vi "0.Main.vi"() -> ()   [LabVIEW 2021]
uses:
  controls/initialise cluster.ctl
  controls/developer_test sequence.ctl
  controls/test step description.ctl
  controls/test type selection.ctl
  controls/comparison selection.ctl
  controls/DMM measuring state.ctl
  <vilib>/Utility/miscctls.llb/LVPointTypeDef.ctl
  support/Message Queue/Enqueue Message (Single).vi
  support/Message Queue/RMU Message Queue.lvlib
  support/User Event - Stop/RMU User Event - Stop.lvlib
  GPT-9800_GSB_L2011/GPT-9000.lvlib
panel:
  out "Output values":T1
  out "Varaint Selection":string
  out "Tempertaure Sensor":string
  out "Result":bool
  out "m second":u32
  out "Hillppot Comport":refnum<visa-resource-name>
  out "Final Weld Resistance Result":string
  out "Limits revision":string
  out "weld voltage":dbl[](array[numeric]) format="%#_6p"
  out "Test Start Time":string
  out "Result indicators":refnum<vi>[](array[refnum])
  out "Limits":string[](array[string])
  out "Current":dbl
  out "Cell 7 - Cell 8 Result":string
  out "Cell 7 - Cell 8":string
  in  "Login Button":bool
  out "login":string
  out "Unlock":bool
  out "Elapsed Time (s)":dbl
  out "stop":bool
  out "Update timer":bool
  out "reset timer":bool
  in  "status_bri":string
  out "weld res":dbl[](array[numeric]) format="%^#.5g"
  out "Temp value":dbl[](array[numeric])
  out "Voltage health check":dbl[](array[numeric])
  out "Array":dbl[](array[numeric])
  out "Cell 8 (End Busbar) Result":string
  out "Cell 6 - Cell 7 Result":string
  out "Cell 5 - Cell 6 Result":string
  out "Final Insulation Resistance Result":string
  out "Final Voltage test result":string
  out "final temp result":string
  out "Cell 4 -Cell 5 Result":string
  out "Cell 3 - Cell 4 Result":string
  out "Cell 2 - Cell 3 Result":string
  out "Cell 1 - Cell 2 Result":string
  out "Cell 1 (End Blusbar) Result":string
  out "Baseplate to Positive Result":string
  out "Baseplate to Negative Result":string
  out "Cell 8S - Voltage Imbalance (mv) Result":string
  out "8S - Voltage Result":string
  out "Min voltage Result":string
  out "Max Voltage Result":string
  out "Cell 8 Result":string
  out "Cell 7 Result":string
  out "Cell 6 Result":string
  out "Cell 5 Result":string
  out "Cell 4 Result":string
  out "Cell 3 Result":string
  out "Cell 2 Result":string
  out "Cell 1 Result":string
  out "Ambient Temperature imbalance Result":string
  out "8S- temperature imbalance Result":string
  out "Min Temperature Result":string
  out "Max Temperature Result":string
  in  "Stop":bool
  in  "Start":bool
  out "Cell 8S - Voltage Imbalance (mv)":string
  out "8S - Voltage":string
  out "Min voltage":string
  out "Max Voltage":string
  out "Cell 8 (End Busbar)":string
  out "Cell 6 - Cell 7":string
  out "Cell 5 - Cell 6":string
  out "Cell 4 -Cell 5":string
  out "Cell 3 - Cell 4":string
  out "Cell 2 - Cell 3":string
  out "Cell 1 - Cell 2":string
  out "Cell 1 (End Blusbar)":string
  out "Baseplate to Positive":string
  out "Baseplate to Negative":string
  out "Cell 8":string
  out "Cell 7":string
  out "Cell 6":string
  out "Cell 5":string
  out "Cell 4":string
  out "Cell 3":string
  out "Cell 2":string
  out "Cell 1":string
  out "Thermistor 4 (Ambient)":string
  out "Thermistor 3":string
  out "Thermistor 2":string
  out "Thermistor 1":string
  out "Ambient Temperature imbalance":string
  out "8S- temperaturen imbalance":string
  out "Min Temperature":string
  out "Max Temperature":string
  out "Status Bar":string
  out "Module Type A/B":string
  out "Module ID":string
  out "Test Duration":string
  # "MODULE EOL"
  # "Application REV-9"
  # "TEST 2 - VOLTAGE HEALTH CHECK"
  # "TEST 3 - INSULATION RESISTANCE TEST"
  # "Insulation\nResistance (Mohm)"
  # "Probing \nPoints"
  # "Result"
  # "Cell No."
  # "Voltage (V)"
  # "Result"
  # "Limits Revision NO"
  # "Baseplate to\nNegative"
  # "Cell 1"
  # "Variant Selection"
  # "Baseplate to\nPositive"
  # "Cell 2"
  # "Temp sensor selection"
  # "Cell 3"
  # "TEST 1 - THERMISTOR HEALTH CHECK"
  # "TEST 4 - WELD RESISTANCE TEST"
  # "Resistance\n  (uohms)"
  # "Thermistor No."
  # "Temperature (C)"
  # "Result"
  # "Probing Points"
  # "Result"
  # "Cell 4"
  # "TEST RESULT SUMMARY"
  # "Cell 1- End Busbar"
  # "Cell 5"
  # "Thermistor 1"
  # "Cell 1 - Cell 2"
  # "Test 1 - THERMISTOR HEALTH CHECK"
  # "Thermistor 2"
  # "Cell 6"
  # "Test 2 - VOLTAGE HEALTH CHECK"
  # "Cell 2 - Cell 3"
  # "Thermistor 3"
  # "Cell 7"
  # "Test 3 - INSULATION RESISTANCE TEST"
  # "Thermistor 4 \n(Ambient)"
  # "Cell 3 - Cell 4"
  # "Cell 8"
  # "Test 4 - WELD RESISTANCE TEST"
  # "Cell 4 - Cell 5"
  # "Max Temperature"
  # "Max Voltage"
  # "Cell 5 - Cell 6"
  # "Min Temperature"
  # "Min Voltage"
  # "Cell 6 - Cell 7"
  # "8S- temperature \nimbalance"
  # "8S - Voltage"
  # "Cell 7 - Cell 8"
  # "Ambient Temperature\nimbalance"
  # "8S - Voltage\nImbalance (mV)"
  # "Cell 8 - End Busbar"
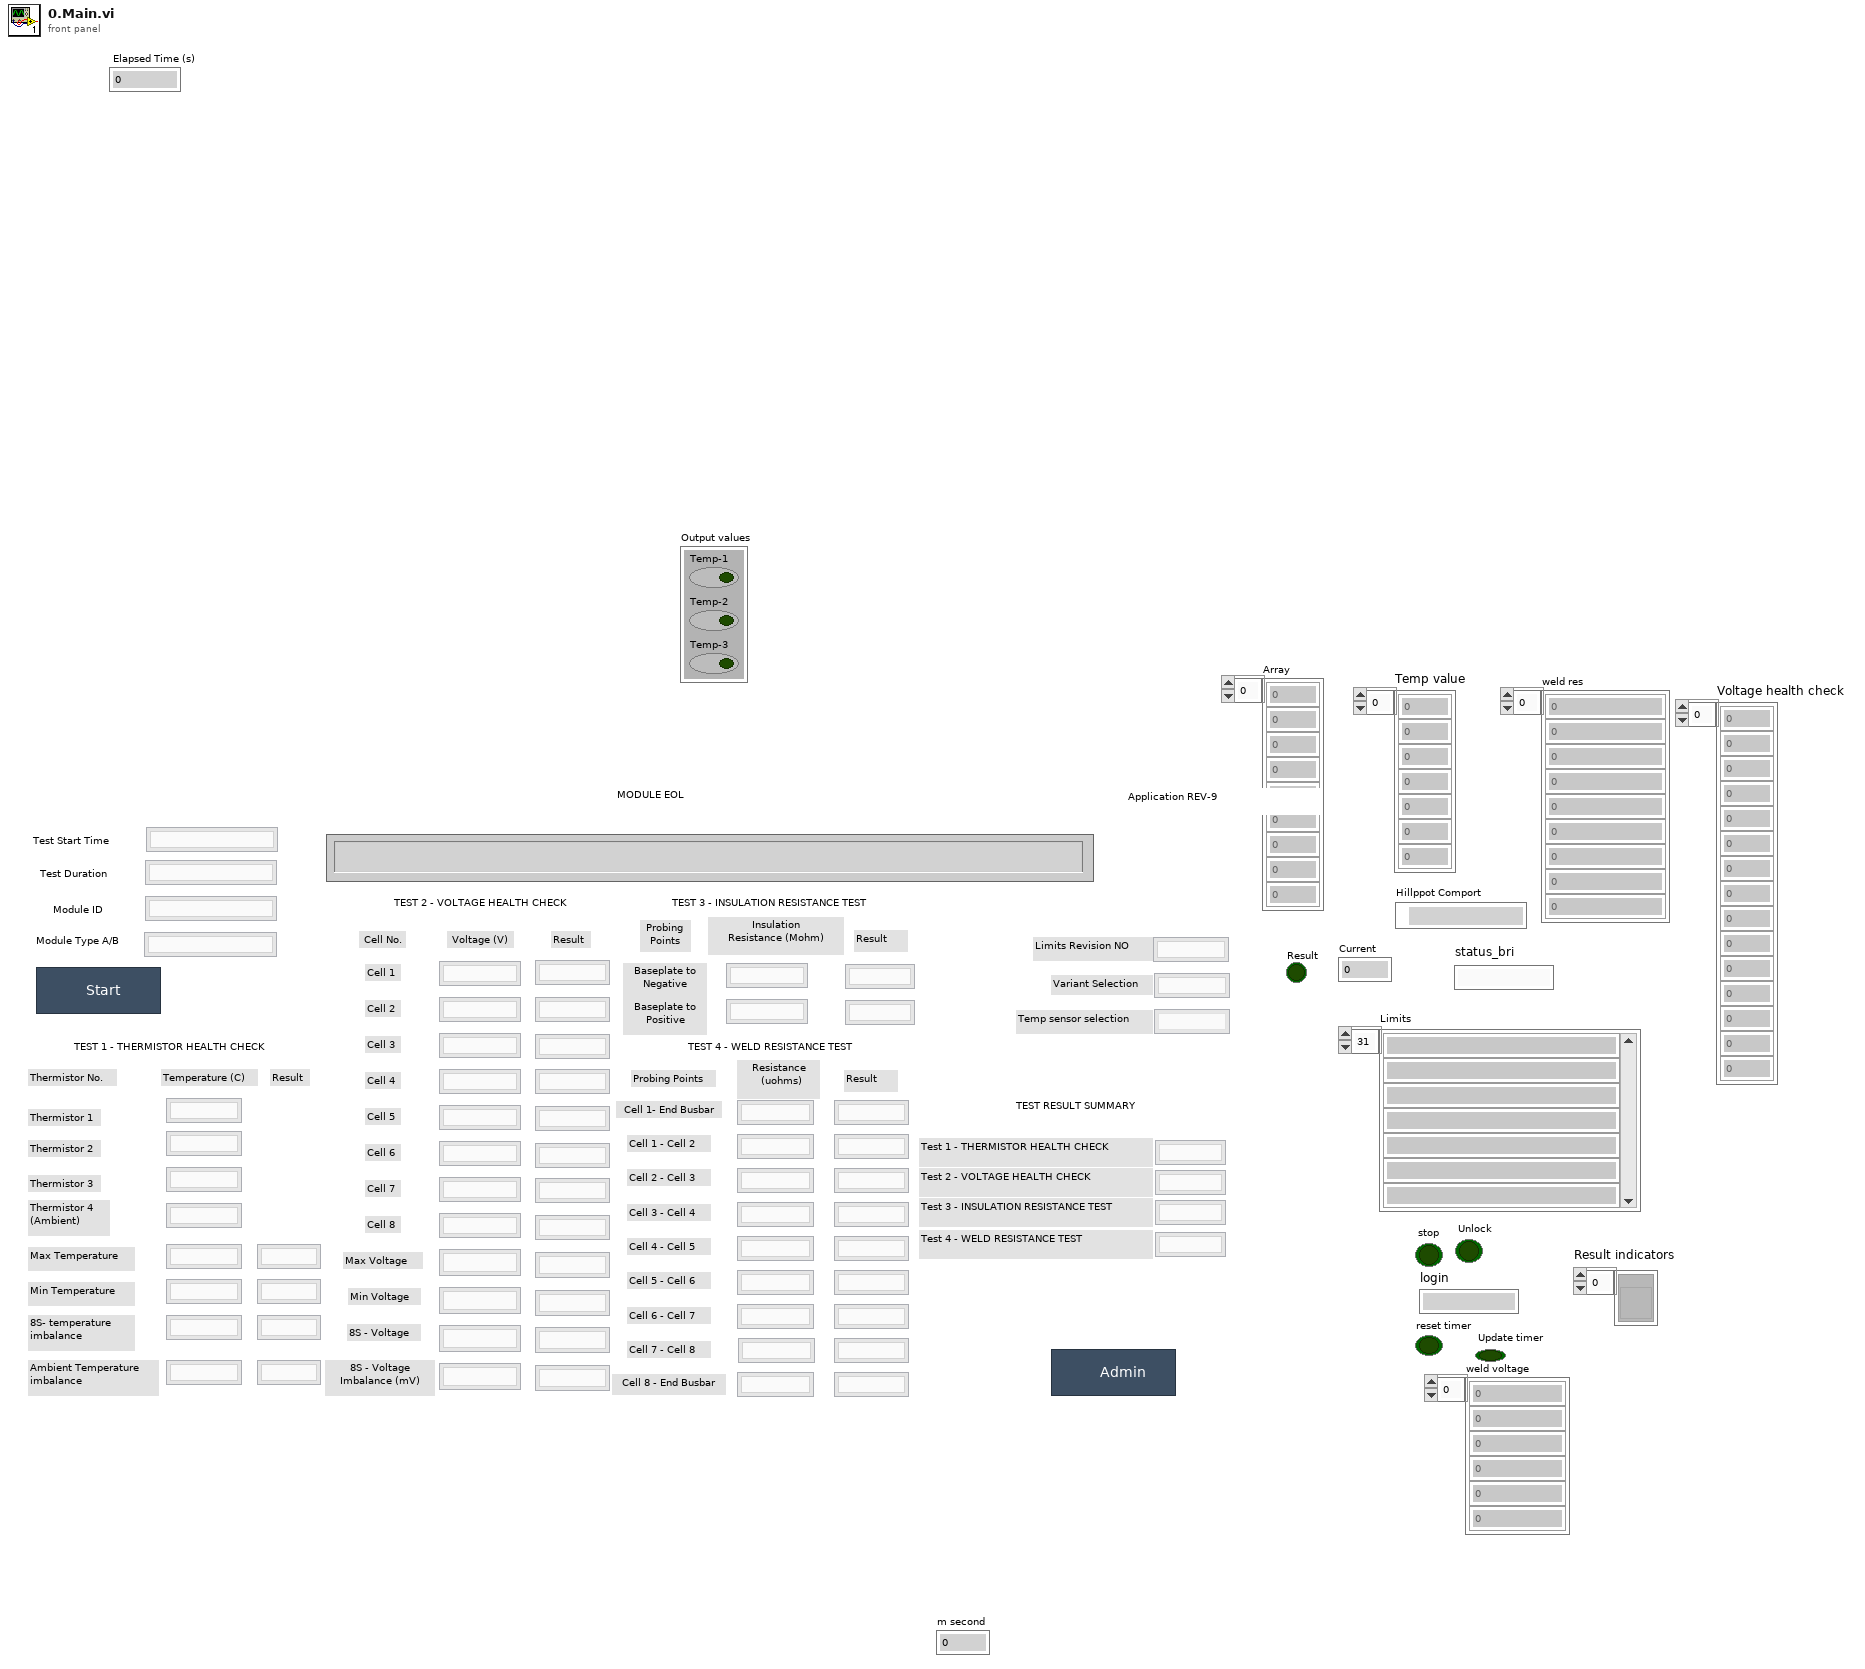
[diagram p1: front panel]
types:
  T1 = cluster{"Temp-1":bool, "Temp-2":bool, "Temp-3":bool}
  T2 = typedef "initialise cluster.ctl" = cluster{"wait value":dbl, "Power supply":refnum<visa-resource-name>, "DMM":refnum<visa-resource-name>, "Arduino":refnum<visa-resource-name>, "RS232 COM5":refnum<visa-resource-name>, "RELAY BOARD":refnum<visa-resource-name>, "test sequence":T3, "Data folder path":path, "user account":string, "test sequence file name":string, "UI":string[][], "DI":T4[], "Skip test?":bool[], "Barcode":string, "DMM measuring state":T7, "T1":string[][], "MCListbox Ref_in":refnum<vi>, "RS232 COM6":refnum<visa-resource-name>, "mains application path":path, "sequence step #":u32, "Screening?":bool, "Result?":bool}
  T3 = typedef "developer_test sequence.ctl" = enum16{"Update Display", "User Login", "Admin", "Initialise", "Init Devices", "Idle State", "test steup", "Abort", "Start Display Board Auto Testing", "Scan Barcode", "Checking TEMP at Thermistor 1", "Checking TEMP at Thermistor 2", "Checking TEMP at Thermistor 3", "Checking TEMP at Thermistor 4 (Ambient)", "Voltage Health Check", "Hillpot connector check", "INSULATION Resistance test (Baseplate to Negative)", "INSULATION Resistance test (Baseplate to Positive)", "Voltage helath check before weld resistance", "Current contactor check", "WELD Resistance Test", "Stop Display Board Auto Testing", "All Pass", "Fail", "Report", "Error", "Confirm Quit", "Exit"}
  T4 = typedef "test step description.ctl" = cluster{"test type":T5, "developer_test sequence":T3, "Lower limit":dbl, "Upper limit":dbl, "Comparison":T6}
  T5 = typedef "test type selection.ctl" = enum16{"None", "Voltage", "Voltage?", "Current", "Current?", "Output", "Program"}
  T6 = typedef "comparison selection.ctl" = enum16{"None", "in-range?", "less than?", "greater than?", "equal to?", "not equal to?", "less or equal to?", "greater or equal to?"}
  T7 = typedef "DMM measuring state.ctl" = u16
  T8 = typedef "RMU Message Queue.lvlib/All Message Queues.ctl" = cluster{"UI":refnum<queue>}
  T9 = typedef "LVPointTypeDef.ctl" = cluster{"Horizontal":i16, "Vertical":i16}
  T10 = enum16{"Weld resistance", "Voltage", "Voltage befor WR", "Temp"}
  T11 = typedef "Control 1.ctl" = string
  T12 = cluster{"Temp sensor out":T11, "Varaint Selection out":string}
  T13 = cluster{"measured value":string, string, "Text.Text Colors:BG Color":u32}[]
  T14 = cluster{"measured value":string, string, "Text.Text Colors:BG Color":u32}
  T15 = cluster{"measured value":string, string, "Status Color":u32}
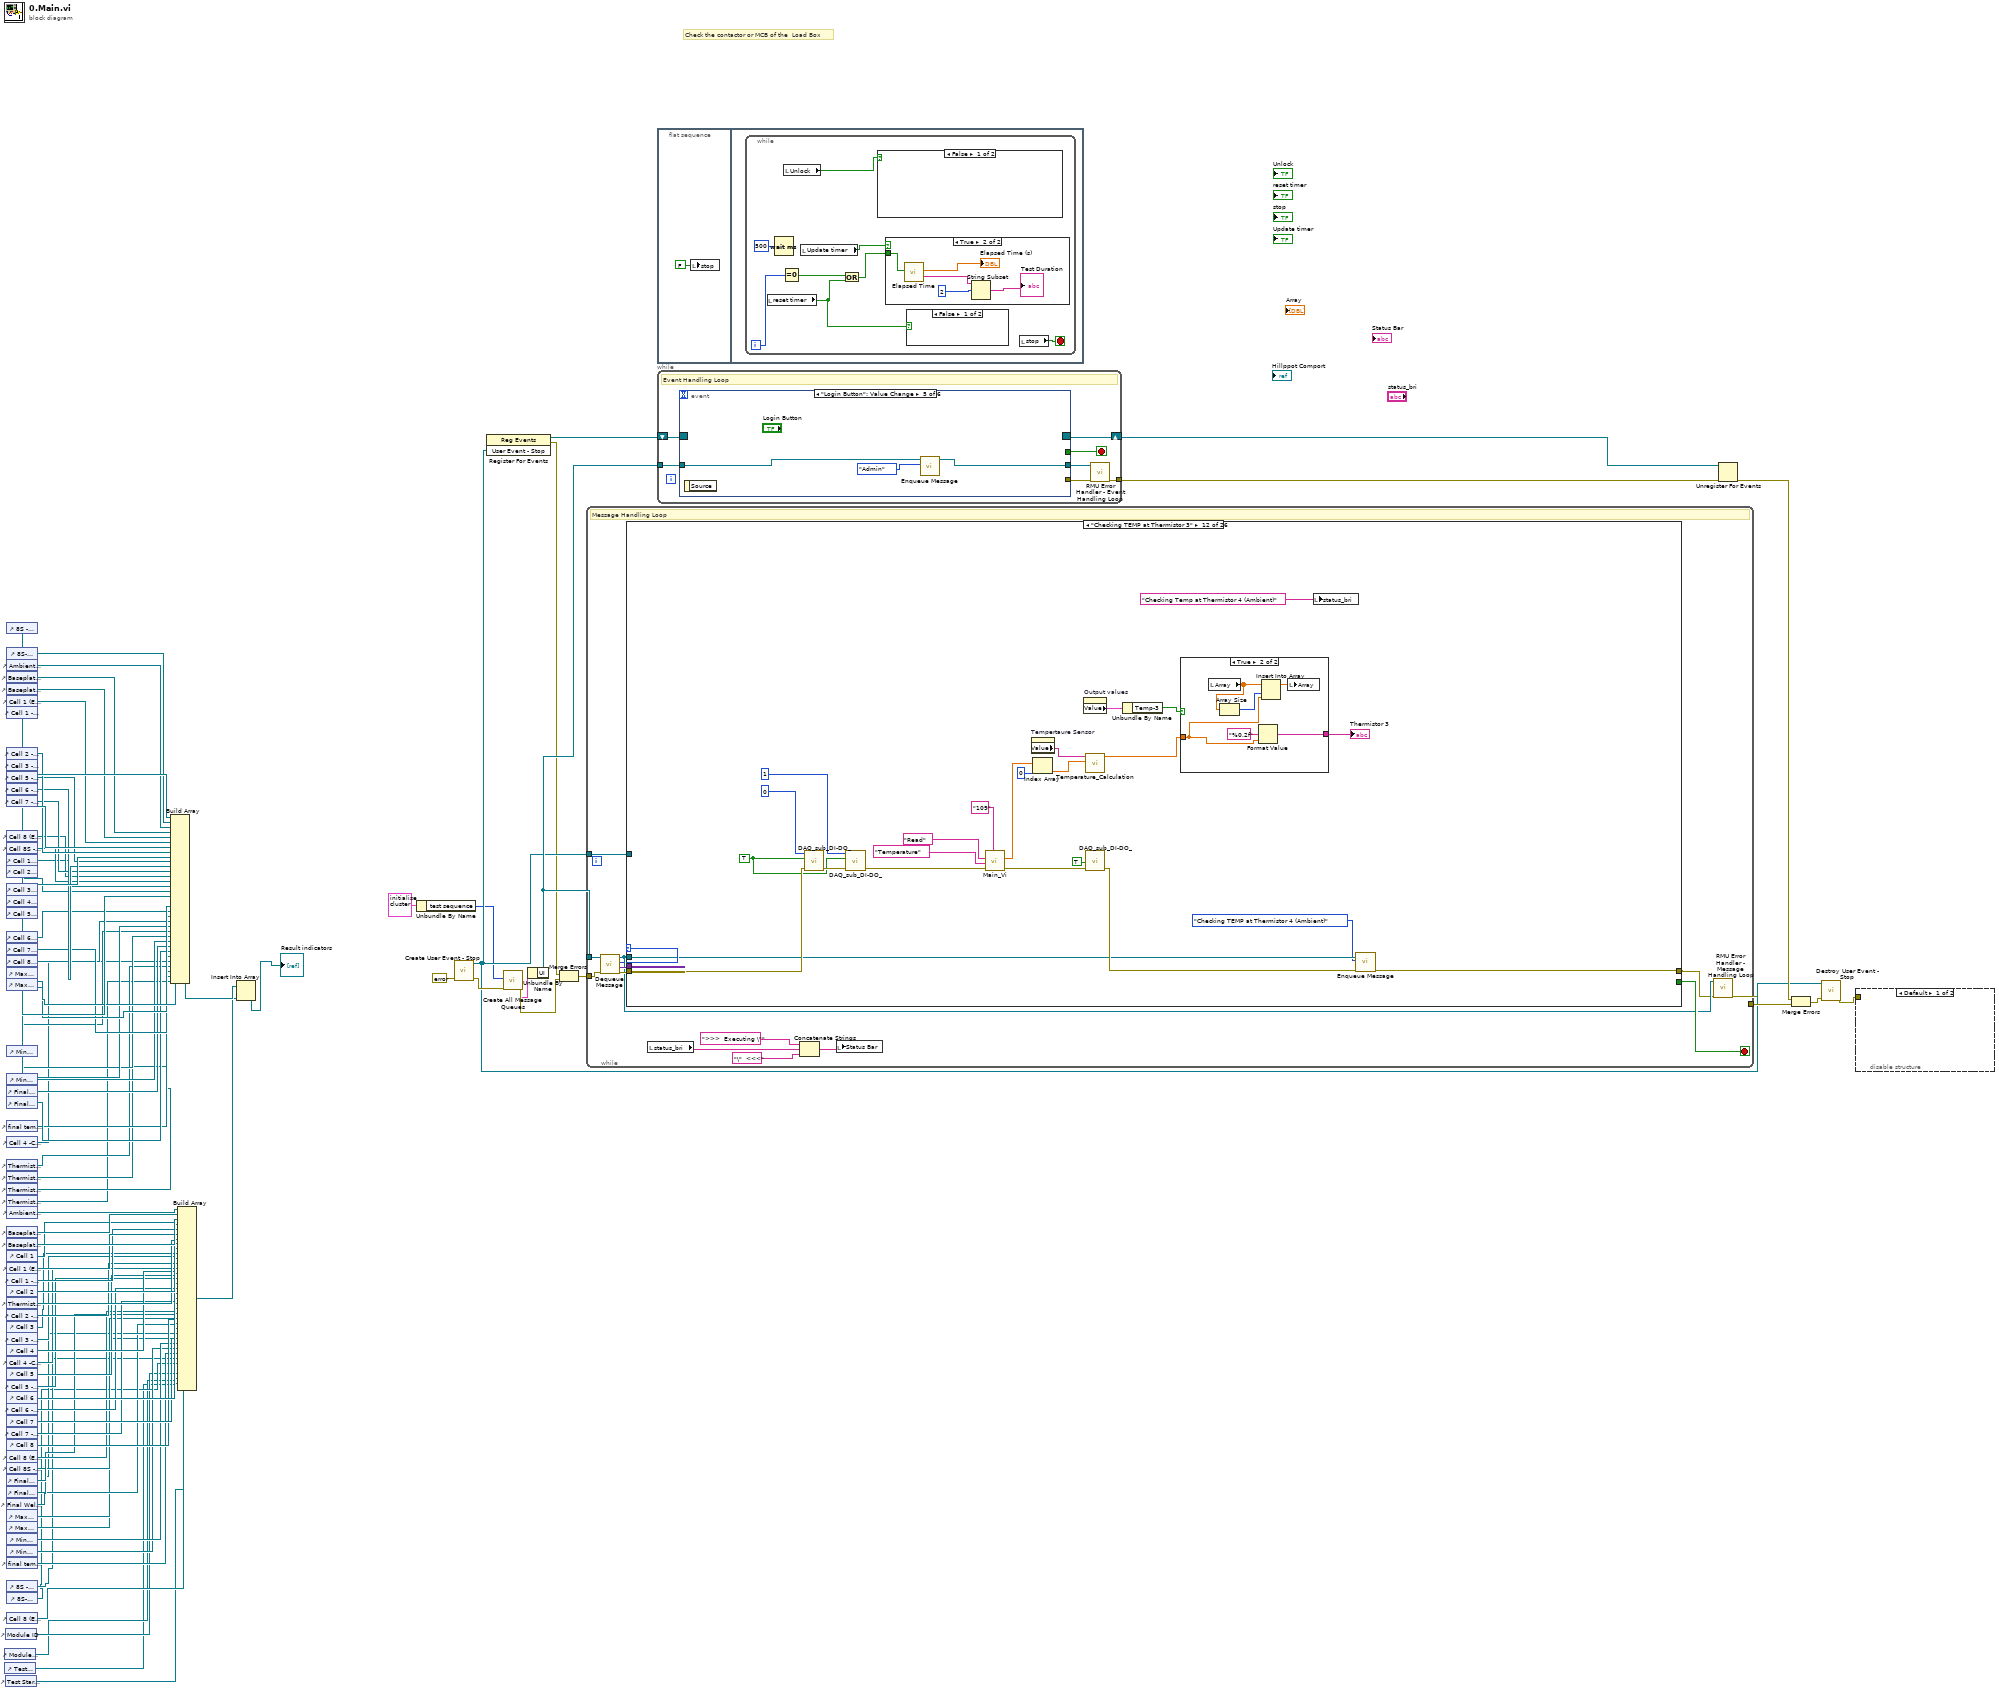
[diagram p0: block diagram]
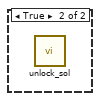
[diagram p2: hidden frame]
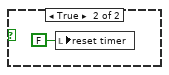
[diagram p3: hidden frame]
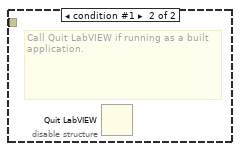
[diagram p5: hidden frame]
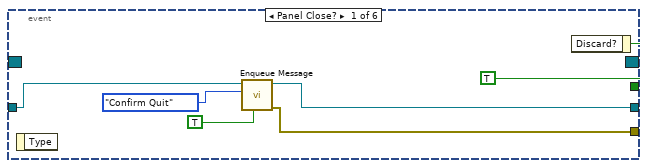
[diagram p6: hidden frame]
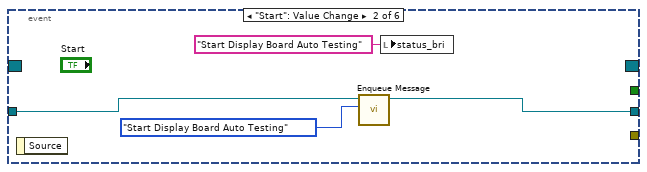
[diagram p7: hidden frame]
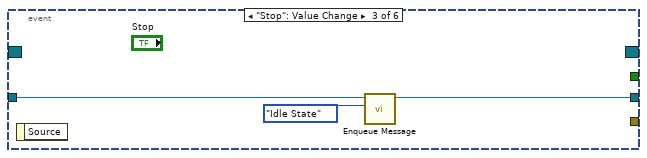
[diagram p8: hidden frame]
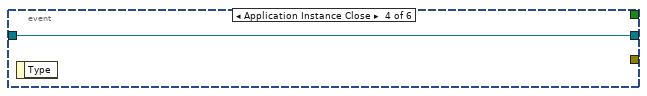
[diagram p9: hidden frame]
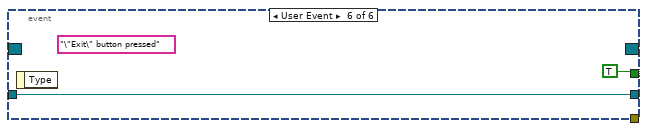
[diagram p10: hidden frame]
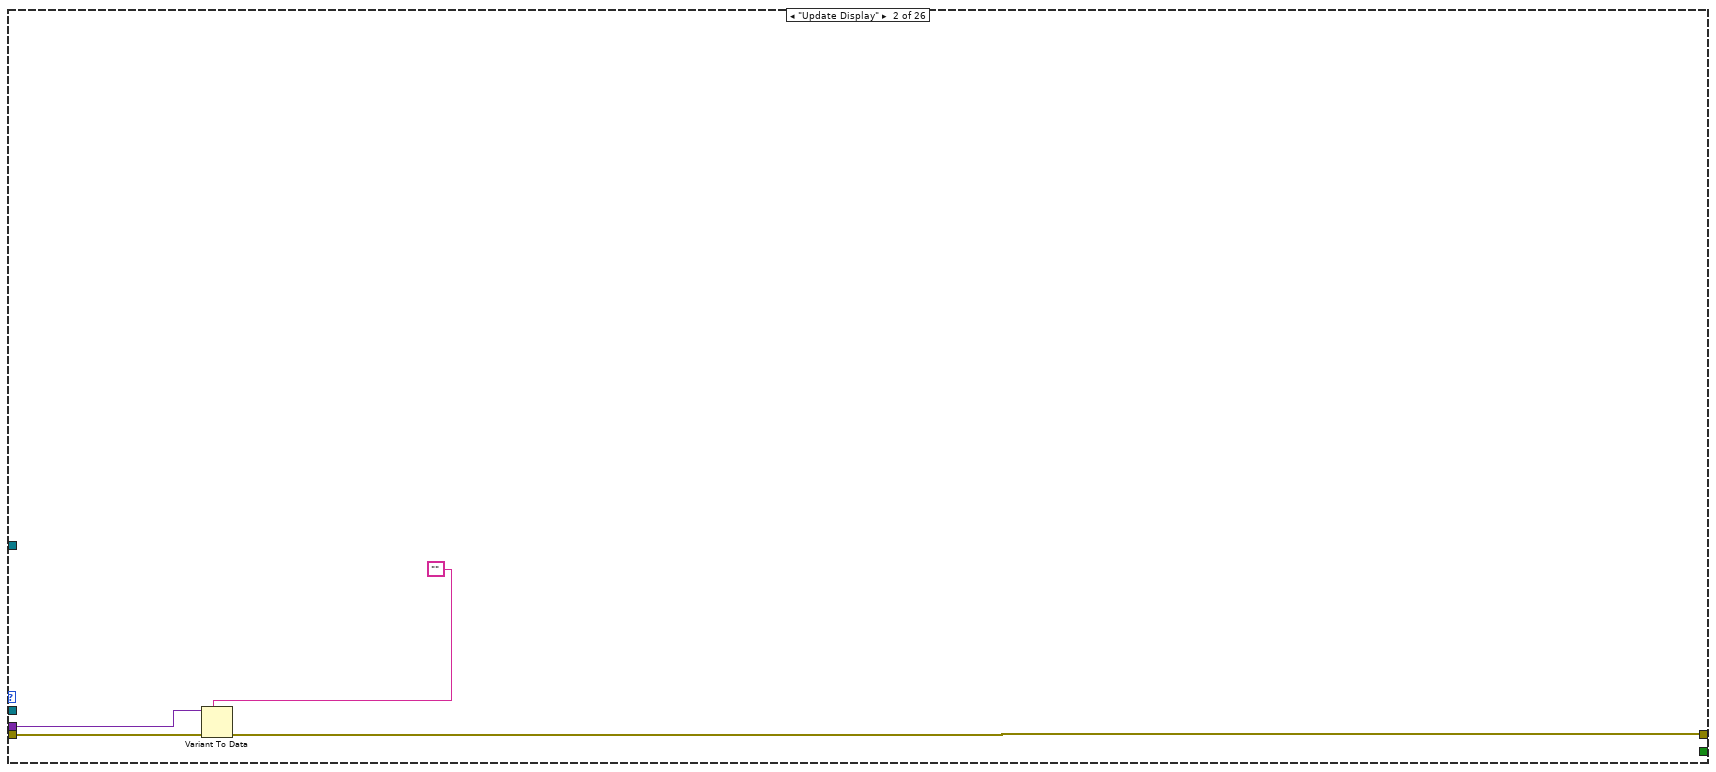
[diagram p12: hidden frame]
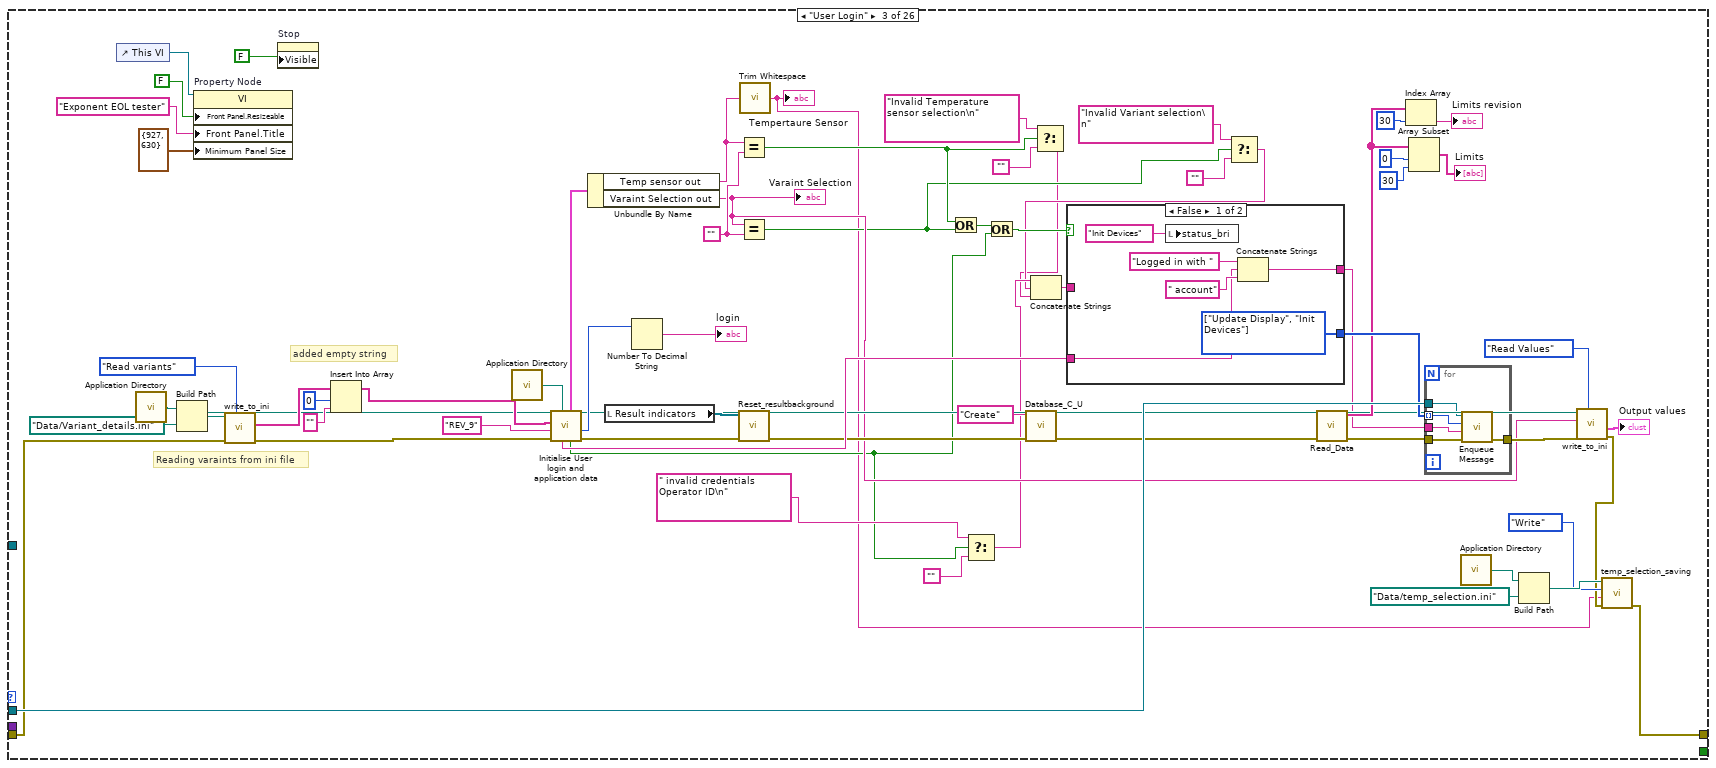
[diagram p13: hidden frame]
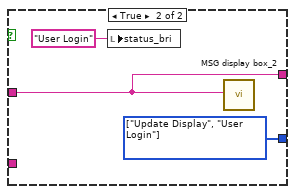
[diagram p14: hidden frame]
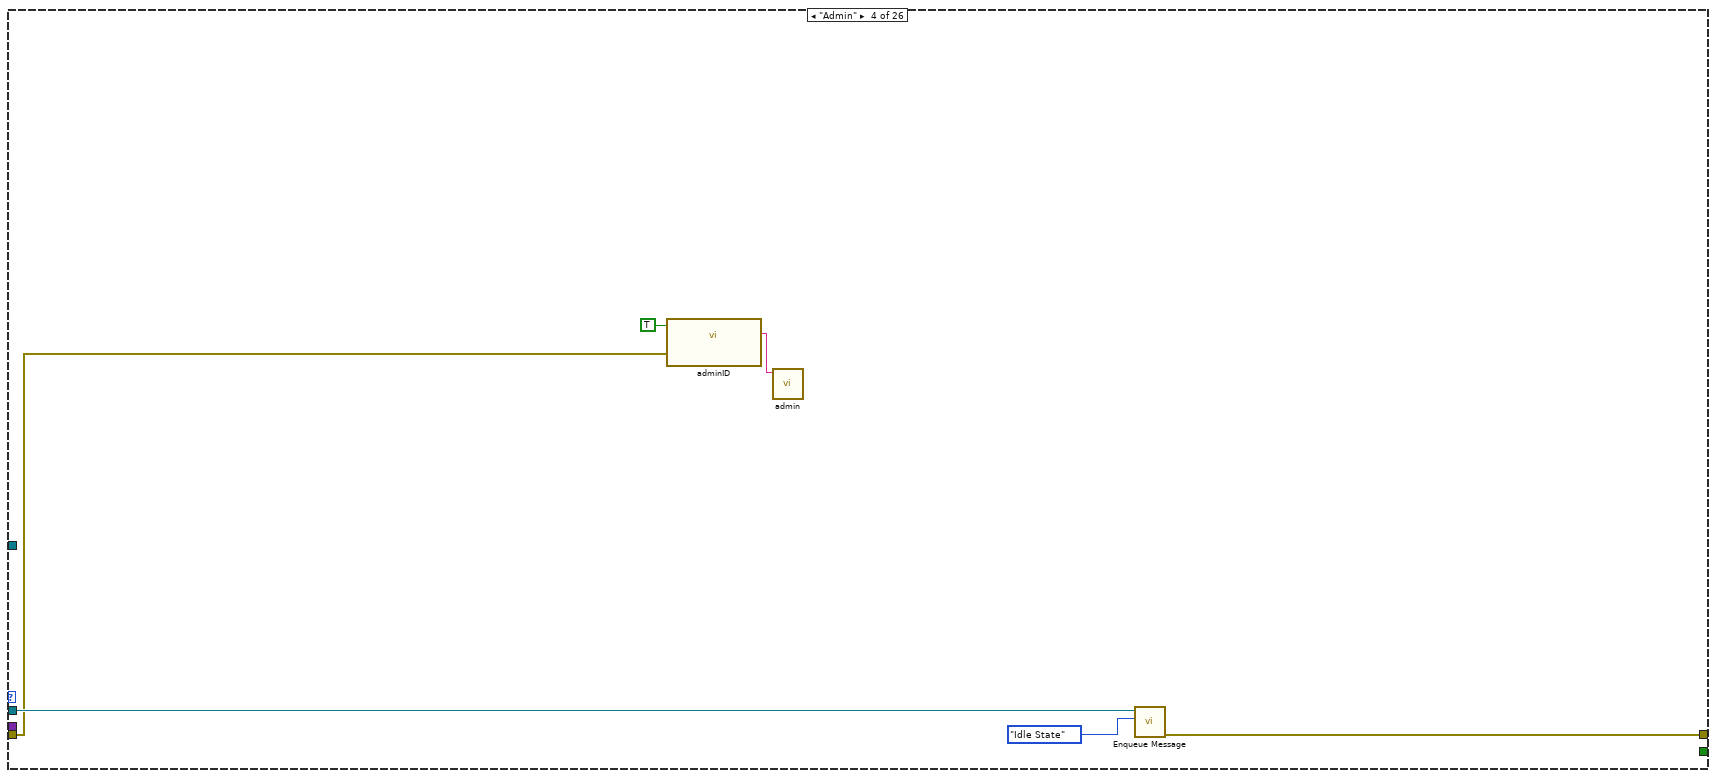
[diagram p15: hidden frame]
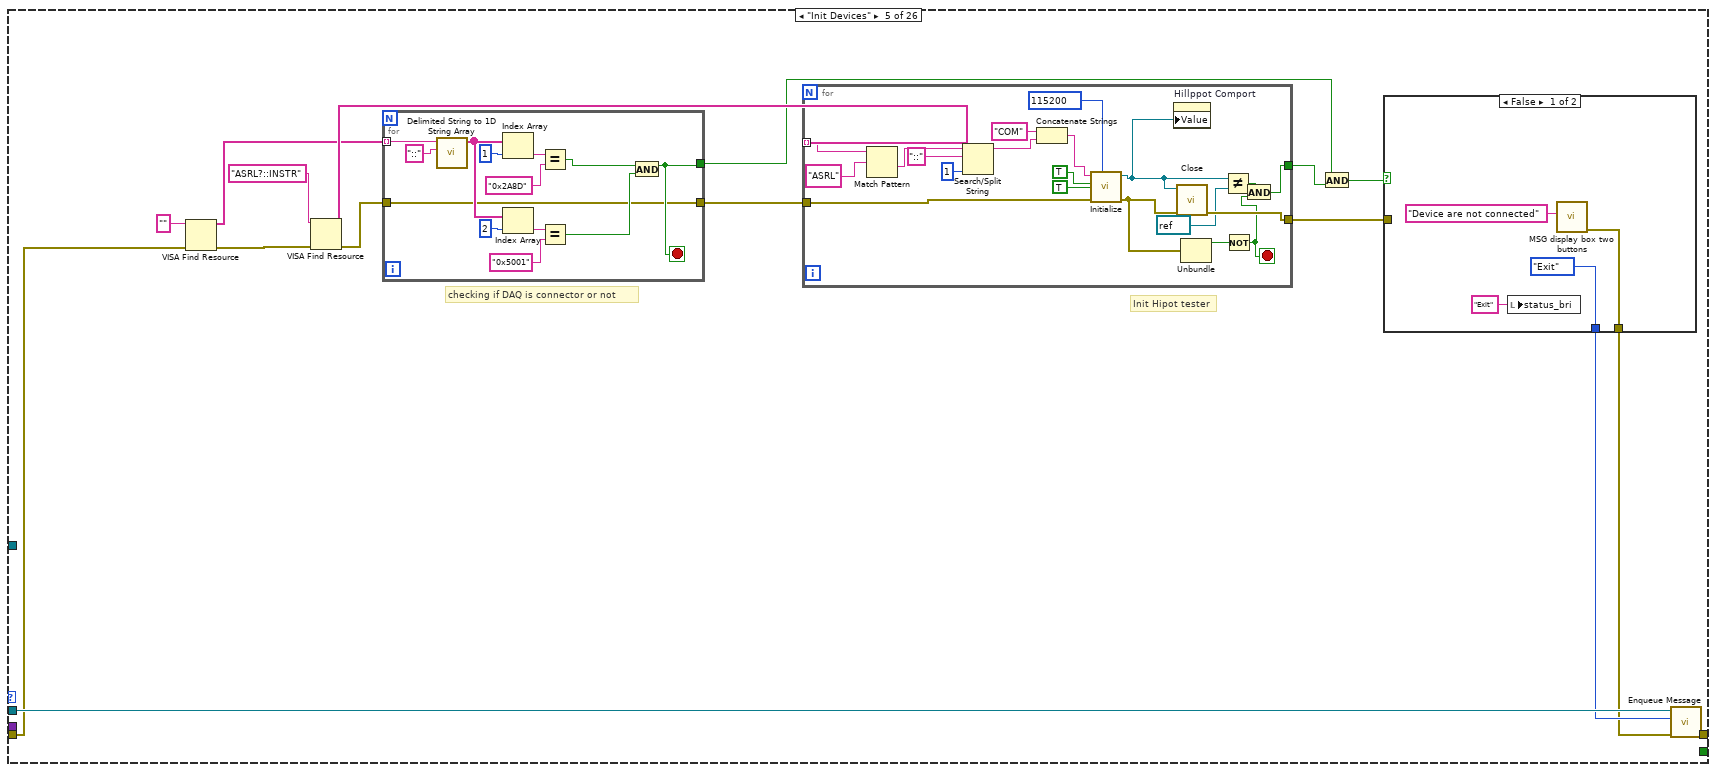
[diagram p16: hidden frame]
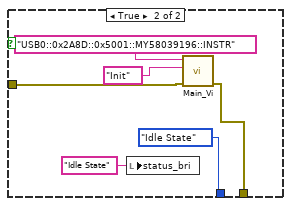
[diagram p17: hidden frame]
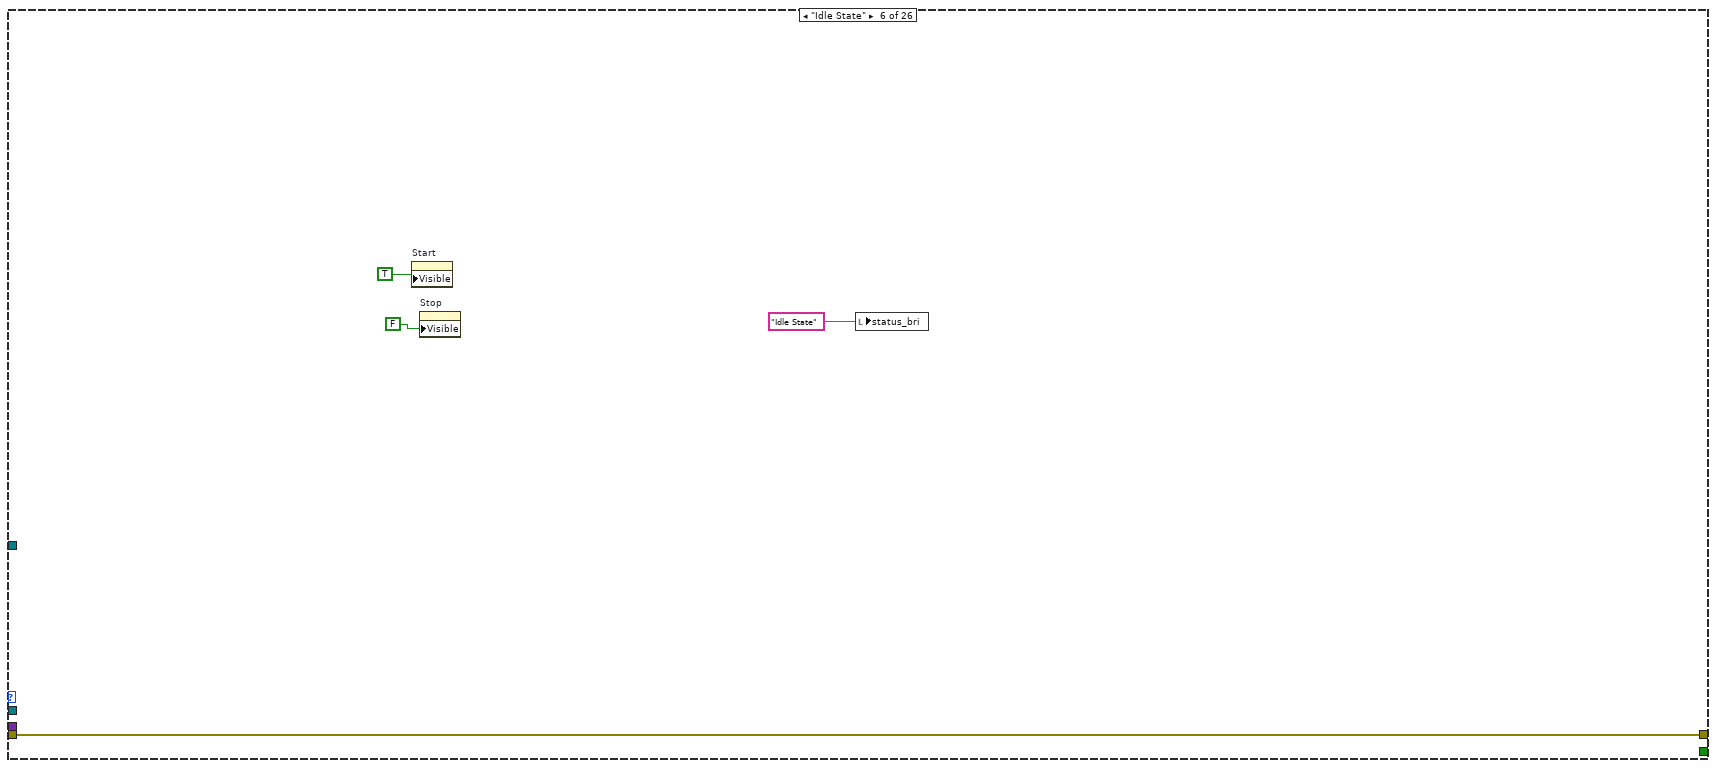
[diagram p18: hidden frame]
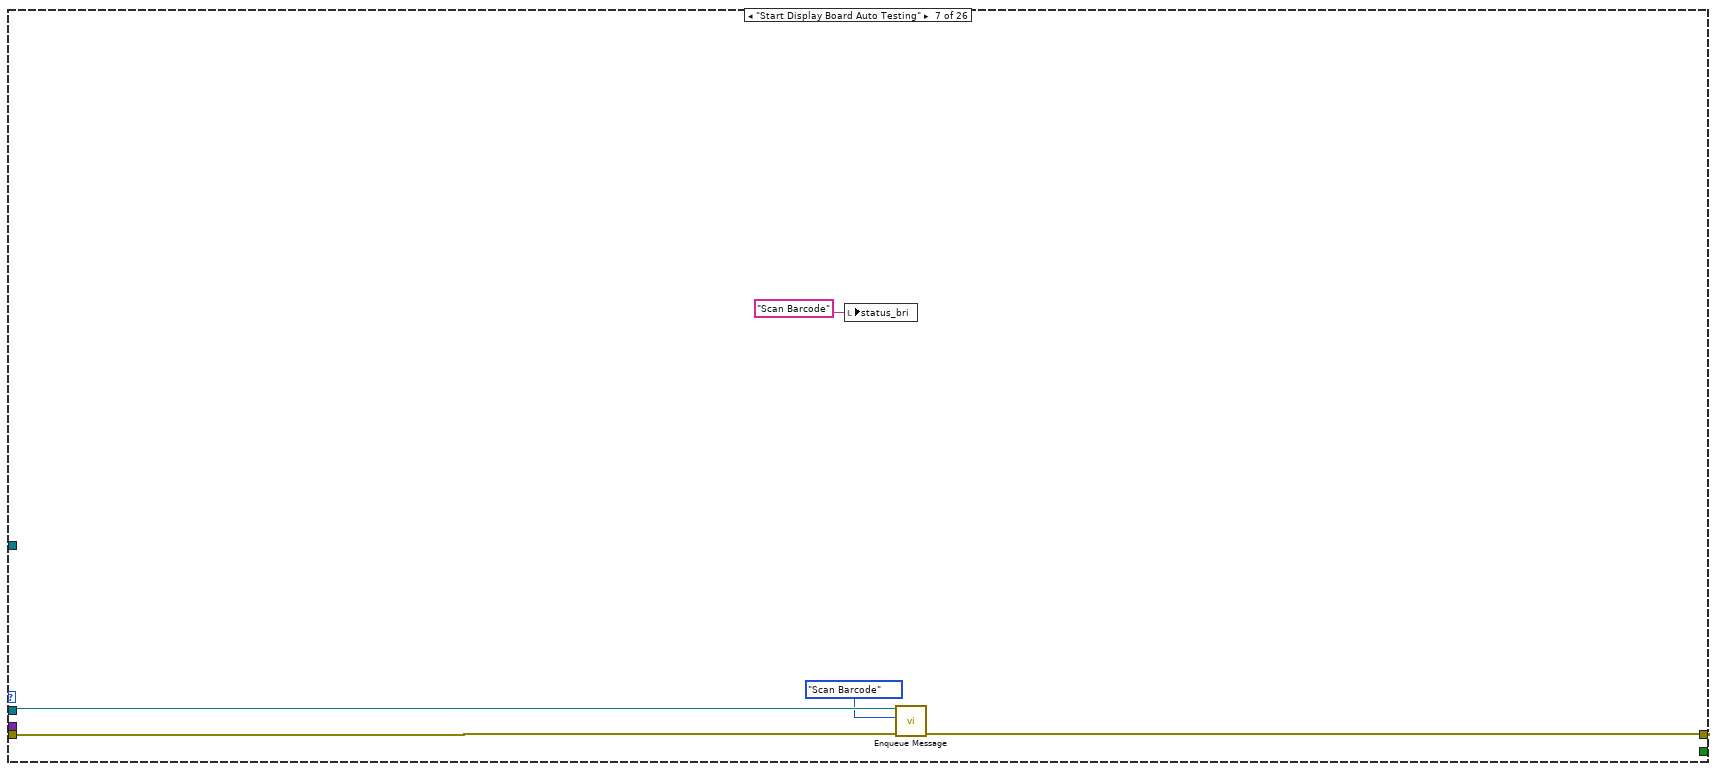
[diagram p19: hidden frame]
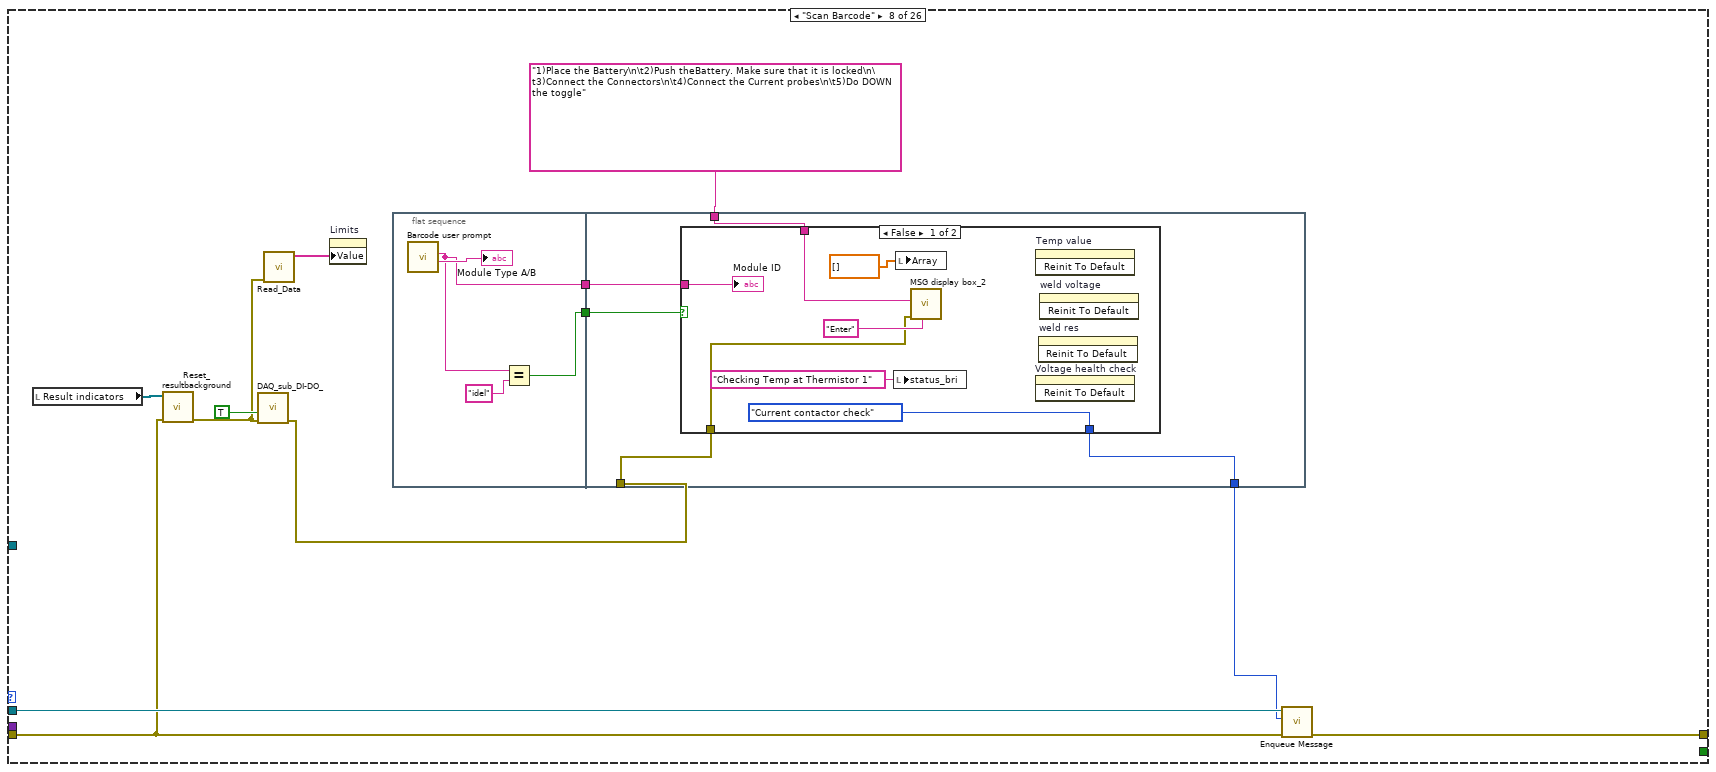
[diagram p20: hidden frame]
diagram:
  # "Check the contactor or MCB of the  Load Box"
  n1 = control-ref of="Module Type A/B"() -> (w3:refnum<vi>)
  n2 = control-ref of="Test Duration"() -> (w2:refnum<vi>)
  n3 = control-ref of="Module ID"() -> (w4:refnum<vi>)
  n4 = control-ref of="Test Start Time"() -> (w1:refnum<vi>)
  n5 = control-ref of="8S - Voltage Result"() -> (w74:refnum<vi>)
  n6 = control-ref of="8S- temperature imbalance Result"() -> (w73:refnum<vi>)
  n7 = control-ref of="Ambient Temperature imbalance Result"() -> (w72:refnum<vi>)
  n8 = control-ref of="Baseplate to Negative Result"() -> (w71:refnum<vi>)
  n9 = control-ref of="Baseplate to Positive Result"() -> (w70:refnum<vi>)
  n10 = control-ref of="Cell 1 (End Blusbar) Result"() -> (w69:refnum<vi>)
  n11 = control-ref of="Cell 1 - Cell 2 Result"() -> (w68:refnum<vi>)
  n12 = control-ref of="Cell 2 - Cell 3 Result"() -> (w67:refnum<vi>)
  n13 = control-ref of="Cell 3 - Cell 4 Result"() -> (w66:refnum<vi>)
  n14 = control-ref of="Cell 5 - Cell 6 Result"() -> (w65:refnum<vi>)
  n15 = control-ref of="Cell 6 - Cell 7 Result"() -> (w64:refnum<vi>)
  n16 = control-ref of="Cell 7 - Cell 8 Result"() -> (w63:refnum<vi>)
  n17 = control-ref of="Cell 8 (End Busbar) Result"() -> (w62:refnum<vi>)
  n18 = control-ref of="Cell 8S - Voltage Imbalance (mv) Result"() -> (w61:refnum<vi>)
  n19 = control-ref of="Cell 1 Result"() -> (w60:refnum<vi>)
  n20 = control-ref of="Cell 2 Result"() -> (w59:refnum<vi>)
  n21 = control-ref of="Cell 3 Result"() -> (w58:refnum<vi>)
  n22 = control-ref of="Cell 4 Result"() -> (w57:refnum<vi>)
  n23 = control-ref of="Cell 5 Result"() -> (w56:refnum<vi>)
  n24 = control-ref of="Cell 6 Result"() -> (w55:refnum<vi>)
  n25 = control-ref of="Cell 7 Result"() -> (w54:refnum<vi>)
  n26 = control-ref of="Cell 8 Result"() -> (w53:refnum<vi>)
  n27 = control-ref of="Max Temperature Result"() -> (w52:refnum<vi>)
  n28 = control-ref of="Max Voltage Result"() -> (w51:refnum<vi>)
  n29 = control-ref of="Min Temperature Result"() -> (w50:refnum<vi>)
  n30 = control-ref of="Min voltage Result"() -> (w49:refnum<vi>)
  n31 = control-ref of="Final Insulation Resistance Result"() -> (w48:refnum<vi>)
  n32 = control-ref of="Final Voltage test result"() -> (w47:refnum<vi>)
  n33 = control-ref of="final temp result"() -> (w46:refnum<vi>)
  n34 = control-ref of="Cell 4 -Cell 5 Result"() -> (w45:refnum<vi>)
  n35 = control-ref of="Thermistor 1"() -> (w44:refnum<vi>)
  n36 = control-ref of="Thermistor 2"() -> (w43:refnum<vi>)
  n37 = control-ref of="Thermistor 3"() -> (w42:refnum<vi>)
  n38 = control-ref of="Thermistor 4 (Ambient)"() -> (w41:refnum<vi>)
  n39 = control-ref of="Ambient Temperature imbalance"() -> (w40:refnum<vi>)
  n40 = control-ref of="Baseplate to Negative"() -> (w39:refnum<vi>)
  n41 = control-ref of="Baseplate to Positive"() -> (w38:refnum<vi>)
  n42 = control-ref of="Cell 1"() -> (w37:refnum<vi>)
  n43 = control-ref of="Cell 1 (End Blusbar)"() -> (w36:refnum<vi>)
  n44 = control-ref of="Cell 1 - Cell 2"() -> (w35:refnum<vi>)
  n45 = control-ref of="Cell 2"() -> (w34:refnum<vi>)
  n46 = control-ref of="Thermistor 4 (Ambient)"() -> (w33:refnum<vi>)
  n47 = control-ref of="Cell 2 - Cell 3"() -> (w32:refnum<vi>)
  n48 = control-ref of="Cell 3"() -> (w31:refnum<vi>)
  n49 = control-ref of="Cell 3 - Cell 4"() -> (w30:refnum<vi>)
  n50 = control-ref of="Cell 4"() -> (w29:refnum<vi>)
  n51 = control-ref of="Cell 4 -Cell 5"() -> (w28:refnum<vi>)
  n52 = control-ref of="Cell 5"() -> (w27:refnum<vi>)
  n53 = control-ref of="Cell 5 - Cell 6"() -> (w26:refnum<vi>)
  n54 = control-ref of="Cell 6"() -> (w25:refnum<vi>)
  n55 = control-ref of="Cell 6 - Cell 7"() -> (w24:refnum<vi>)
  n56 = control-ref of="Cell 7"() -> (w23:refnum<vi>)
  n57 = control-ref of="Cell 7 - Cell 8"() -> (w22:refnum<vi>)
  n58 = control-ref of="Cell 8"() -> (w21:refnum<vi>)
  n59 = control-ref of="Cell 8 (End Busbar) Result"() -> (w20:refnum<vi>)
  n60 = control-ref of="Cell 8S - Voltage Imbalance (mv)"() -> (w18:refnum<vi>)
  n61 = control-ref of="Final Insulation Resistance Result"() -> (w19:refnum<vi>)
  n62 = control-ref of="Final Voltage test result"() -> (w16:refnum<vi>)
  n63 = control-ref of="Final Weld Resistance Result"() -> (w17:refnum<vi>)
  n64 = control-ref of="Max Temperature"() -> (w15:refnum<vi>)
  n65 = control-ref of="Max Voltage"() -> (w14:refnum<vi>)
  n66 = control-ref of="Min Temperature"() -> (w13:refnum<vi>)
  n67 = control-ref of="Min voltage"() -> (w12:refnum<vi>)
  n68 = control-ref of="final temp result"() -> (w11:refnum<vi>)
  n69 = control-ref of="8S - Voltage"() -> (w7:refnum<vi>)
  n70 = control-ref of="8S- temperaturen imbalance"() -> (w6:refnum<vi>)
  n71 = control-ref of="Cell 8 (End Busbar)"() -> (w5:refnum<vi>)
  n72 = Build Array(w74, w73, w72, w71, w70, w69, w68, w67, w66, w65, w64, w63, w62, w61, w60, w59, w58, w57, w56, w55, w54, w53, w52, w51, w50, w49, w48, w47, w46, w45, w44, w43, w42, w41) -> (w10:refnum<vi>[])
  n73 = Build Array(w40, w39, w38, w37, w35, w36, w33, w34, w32, w31, w30, w29, w28, w27, w26, w25, w24, w23, w22, w21, w20, w19, w18, w16, w17, w15, w14, w13, w12, w11, w7, w6, w5, w4, w3, w2, w1) -> (w9:refnum<vi>[])
  n74 = Insert Into Array(array=w10, new element=w9) -> (→"Result indicators":refnum<vi>[])  [unwired: 1 in]
  n75 = Unbundle By Name(T2 {"wait value"=0.0, "Power supply"="COM1", "DMM"="COM1", "Arduino"="COM1", "RS232 COM5"="COM1", "RELAY BOARD"="COM1", "test sequence"=enum."User Login", "Data folder path"=path "", "user account"="", "test sequence file name"="", "UI"=[], "DI"=[], "Skip test?"=[FALSE, FALSE, FALSE, FALSE, FALSE, FALSE, FALSE, FALSE, FALSE, FALSE, FALSE, FALSE, FALSE, FALSE, FALSE, FALSE, FALSE, FALSE, FALSE, FALSE, FALSE, FALSE, FALSE, FALSE, FALSE, FALSE, FALSE, FALSE, FALSE, FALSE, FALSE, FALSE], "Barcode"="", "DMM measuring state"=2, "T1"=[], "MCListbox Ref_in"=refnum, "RS232 COM6"="COM1", "mains application path"=path "", "sequence step #"=0, "Screening?"=FALSE, "Result?"=FALSE} ("Initialise cluster")) -> ("test sequence"=w77:T3)
  n76 = call "Create User Event - Stop.vi"("error in (no error)"=errorcluster {"status"=FALSE, "code"=0, "source"=""}) -> ("error out"=w87:errorcluster, "User Event - Stop"=w80:refnum<user-event>)  [unwired: 9 in]
  n77 = register-events(w80) -> (reference out=w81:refnum<event-registration>, error out=w78:errorcluster)  [unwired: 2 in]
  n78 = call "Create All Message Queues.vi"("error in (no error)"=w87, "test sequence"=w77) -> ("error out"=w91:errorcluster, "Message Queues out"=w90:T8)  [unwired: 8 in]
  n79 = Unbundle By Name(w90) -> ("UI"=w88:refnum<queue>)
  n80 = Merge Errors(w78, w91) -> (w79:errorcluster)
  n81 = while {
    tunnel: w88 -> [w100]
    tunnel: w80 -> [w104]
    tunnel: w79 -> [w103]
    tunnel: [w98] -> w89
    stop <- w105 stop-if-true
    # "Message Handling Loop"
    n82 = call "Dequeue Message.vi"("error in (no error)"=w103, "Message Queue"=w100) -> ("error out"=w102:errorcluster, "Message Data"=w101:variant, "developer_test sequence"=w94:T3, "dup Message Queue"=w99:refnum<queue>)  [unwired: 6 in]
    n83 = case "Message Cases" shown="\"Checking TEMP at Thermistor 3\"" w94 {
      tunnel: w99 -> [_ _ w174 w194 w209 _ w262 w274 w309 w334 w365 w396 w466 w567 w616 w650 w691 w732 w835 w846 w869 w970 _ w1002 w1016 _]
      tunnel: w102 -> [w106 w110 w137 w191 w196 w257 w260 w270 w305 w323 w373 w404 w472 w597 w619 w656 w696 w738 w791 _ w867 w966 w997 w1005 w1011 w1020]
      tunnel: [w106 w107 w112 w193 w210 w257 w261 w273 w310 w332 w362 w398 w467 w569 w615 w649 w677 w734 w834 w847 w868 w891 w992 w1004 w1009 w1020] -> w97
      tunnel: [_ _ _ _ _ _ _ _ _ _ _ _ _ _ _ _ _ _ _ _ _ _ _ _ TRUE _] -> w105
      tunnel: w101 -> [_ w109 _ _ _ _ _ _ _ _ _ _ _ _ _ _ _ _ _ _ _ _ w996 _ w1010 _]
      tunnel: w104 -> [_ _ _ _ _ _ _ _ _ _ _ _ _ _ _ _ _ _ _ _ _ _ _ _ w1013 _]
      frame Default {
        # "'Default' case only runs if there is a message that isn't defined in any of the other cases.  Output a programming error."
      }
      frame "Update Display" {
        # "Update Display - Convert the message data to a string to display in the Data Display indicator."
        n84 = Variant To Data(error in=w110, type="", Variant=w109) -> (error out=w107:errorcluster)  [unwired: 1 out]
      }
      frame "User Login" {
        w142 = ""
        # "added empty string"
        # "Reading varaints from ini file"
        # "Login window"
        n85 = control-ref of="This VI"() -> (w168:refnum<vi>)
        n86 = call <vilib>:"Application Directory.vi"() -> ("Application Directory"=w149:path)
        n87 = Build Path(base path=w149, name or relative path=path "Data/Variant_details.ini") -> (appended path=w134:path)
        n88 = property on="Property Node" class="VI"(reference=w168, "Front Panel.Resizeable"=FALSE ("Front Panel Window:Resizable"), "Front Panel.Title"="Exponent EOL tester" ("Front Panel Window:Title"), "Minimum Panel Size"=T9 {"Horizontal"=927, "Vertical"=630} ("Front Panel Window:Minimum Size")) -> ()  [unwired: 1 in, 2 out]
        n89 = call "write_to_ini.vi"("Enum"=enum16{"Write", "Read variants", "Read Values"}."Read variants", "error in (no error)"=w137, "configuration file path"=w134) -> ("error out"=w136:errorcluster, "section names"=w145:string[])  [unwired: 5 in, 2 out]
        n90 = property on="Stop" class="Bool"("Visible"=FALSE) -> ()  [unwired: 2 in, 2 out]
        n91 = Insert Into Array(array=w145, index=0, new element="" ("new element/subarray")) -> (w146:string[])
        n92 = call <vilib>:"Application Directory.vi"() -> ("Application Directory"=w171:path)
        n93 = call "Initialise User login and application data.vi"("mains application path"=w171, "error in"=w136, "Revision number"="REV_9", "Strings []"=w146) -> ("error out"=w160:errorcluster, "User name"=w156:i32, "Stop App?"=w123:bool, "Varient&temp"=w150:T12, "selected account name"=w172:string)  [unwired: 1 in, 2 out]
        n94 = Unbundle By Name(w150) -> ("Temp sensor out"=w139:T11, "Varaint Selection out"=w132:string)
        "Varaint Selection" <- w132
        n95 = local read "Result indicators"() -> (w159:refnum<vi>[])
        n96 = Number To Decimal String(number=w156) -> (decimal integer string=→"login":string)  [unwired: 1 in]
        n97 = Equal?(x=w139, y=w142) -> (x = y?=w131:bool)
        n98 = Equal?(x=w132, y=w142) -> (x = y?=w126:bool)
        n99 = call "Reset_resultbackground.vi"("error in (no error)"=w160, "appended array"=w159) -> ("error out"=w161:errorcluster)  [unwired: 9 in]
        n100 = call <vilib>:"Trim Whitespace.vi"("string"=w139) -> ("trimmed string"=w111:string)  [unwired: 1 in]
        "Tempertaure Sensor" <- w111
        n101 = Or(x=w131, y=w126) -> (x .or. y?=w140:bool)
        n102 = Select(t=" invalid credentials Operator ID\n", s=w123, f="") -> (s? t:f=w122:string)
        n103 = Or(x=w140, y=w123) -> (x .or. y?=w141:bool)
        n104 = call "Database_C_U.vi"("error in (no error)"=w161, "Combo Box"="Create") -> ("error out"=w163:errorcluster)  [unwired: 8 in, 1 out]
        n105 = Select(t="Invalid Temperature sensor selection\n", s=w131, f="") -> (s? t:f=w120:string)
        n106 = Select(t="Invalid Variant selection\n", s=w126, f="") -> (s? t:f=w121:string)
        n107 = Concatenate Strings(w122, w121, w120) -> (w119:string)
        n108 = case shown="False" w141 {
          tunnel: w172 -> [w183 _]
          tunnel: [w182 w188] -> w173
          tunnel: [w181 w186] -> w118
          tunnel: w119 -> [_ w186]
          frame False {
            w182 = T3[] [enum."Update Display", enum."Init Devices"] items=["Update Display", "User Login", "Admin", "Initialise", "Init Devices", "Idle State", "test steup", "Abort", "Start Display Board Auto Testing", "Scan Barcode", "Checking TEMP at Thermistor 1", "Checking TEMP at Thermistor 2", "Checking TEMP at Thermistor 3", "Checking TEMP at Thermistor 4 (Ambient)", "Voltage Health Check", "Hillpot connector check", "INSULATION Resistance test (Baseplate to Negative)", "INSULATION Resistance test (Baseplate to Positive)", "Voltage helath check before weld resistance", "Current contactor check", "WELD Resistance Test", "Stop Display Board Auto Testing", "All Pass", "Fail", "Report", "Error", "Confirm Quit", "Exit"]
            n109 = local write "status_bri"("Init Devices" ("status_bri")) -> ()
            n110 = Concatenate Strings("Logged in with " ("\"Do Something\" button pressed"), w183, " account" ("string")) -> (w181:string)
          }
          frame True {
            w188 = T3[] [enum."Update Display", enum."User Login"] items=["Update Display", "User Login", "Admin", "Initialise", "Init Devices", "Idle State", "test steup", "Abort", "Start Display Board Auto Testing", "Scan Barcode", "Checking TEMP at Thermistor 1", "Checking TEMP at Thermistor 2", "Checking TEMP at Thermistor 3", "Checking TEMP at Thermistor 4 (Ambient)", "Voltage Health Check", "Hillpot connector check", "INSULATION Resistance test (Baseplate to Negative)", "INSULATION Resistance test (Baseplate to Positive)", "Voltage helath check before weld resistance", "Current contactor check", "WELD Resistance Test", "Stop Display Board Auto Testing", "All Pass", "Fail", "Report", "Error", "Confirm Quit", "Exit"]
            n111 = local write "status_bri"("User Login" ("status_bri")) -> ()
            n112 = call "MSG display box_2.vi"("input string"=w186) -> ()  [unwired: 8 in, 3 out]
          }
        }
        n113 = call "Read_Data.vi"("error in"=w163) -> ("error out"=w162:errorcluster, "string array"=w151:string[])  [unwired: 9 in]
        n114 = Index Array(array=w151, index=30) -> (element=→"Limits revision":string)
        n115 = Array Subset(array=w151, index=0, length=30) -> (→"Limits":string[])
        n116 = for {
          tunnel: w173 -> [w179] mode=indexing
          tunnel: w174 -> [w178]
          tunnel: w162 -> [w177]
          tunnel: [w176] -> w135
          tunnel: w118 -> [w175]
          n117 = call-poly "Enqueue Message.vi"("error in (no error)"=w177, "Message Data"=w175, "test sequence"=w179, "Message Queue"=w178) -> ("error out"=w176:errorcluster)  [unwired: 6 in, 1 out]
        }
        n118 = call <vilib>:"Application Directory.vi"() -> ("Application Directory"=w116:path)
        n119 = Build Path(base path=w116, name or relative path=path "Data/temp_selection.ini") -> (appended path=w117:path)
        n120 = call "write_to_ini.vi"("Enum"=enum16{"Write", "Read variants", "Read Values"}."Read Values", "error in (no error)"=w135, "String"=w132, "configuration file path"=w134) -> ("error out"=w113:errorcluster, "Output values"=→"Output values":T1)  [unwired: 4 in, 2 out]
        n121 = call "temp_selection_saving.vi"("error in (no error)"=w113, "temp selection"=w111, "Enum"=enum16{"Write", "Read Values"}."Write", "configuration file path"=w117) -> ("error out"=w112:errorcluster)  [unwired: 5 in, 2 out]
      }
      frame "Admin" {
        n122 = call "adminID.vi"("Enable"=TRUE, "error in (no error)"=w191) -> ("Operator ID"=w189:string)  [unwired: 15 in, 2 out]
        n123 = call "admin.vi"("Password"=w189) -> ()  [unwired: 11 in]
        n124 = call-poly "Enqueue Message.vi"("test sequence"=developer_test_sequence."Idle State", "Message Queue"=w194) -> ("error out"=w193:errorcluster)  [unwired: 8 in, 1 out]
      }
      frame "Init Devices" {
        # "Init Hipot tester"
        # "checking if DAQ is connector or not"
        # "Initialize - All initialization work should take place in this message, since other loops can potentially enqueue messages that execute immediately after this one."
        n125 = VISA Find Resource(8:w196, 11:"" ("expression (\"?*\")")) -> (0:w195:errorcluster, 3:w197:string[])  [unwired: 1 in, 1 out]
        n126 = VISA Find Resource(8:w195, 11:"ASRL?::INSTR" ("expression (\"?*\")")) -> (0:w204:errorcluster, 3:w206:string[])  [unwired: 1 in, 1 out]
        n127 = for {
          tunnel: w197 -> [w243] mode=indexing
          tunnel: [w232] -> w201
          tunnel: [w231] -> w205
          tunnel: w204 -> [w231]
          stop <- w232 stop-if-true
          n128 = call <vilib>:"Delimited String to 1D String Array.vi"("delimiter"="::" ("search string/char (-)"), "delimited string"=w243) -> ("string array"=w241:string[])  [unwired: 9 in]
          n129 = Index Array(array=w241, index=1) -> (element=w238:string)
          n130 = Index Array(array=w241, index=2) -> (element=w237:string)
          n131 = Equal?(x=w238, y="0x2A8D") -> (x = y?=w234:bool)
          n132 = Equal?(x=w237, y="0x5001") -> (x = y?=w233:bool)
          n133 = And(x=w234, y=w233) -> (x .and. y?=w232:bool)
        }
        n134 = for {
          tunnel: w206 -> [w220] mode=indexing
          tunnel: w205 -> [w228]
          tunnel: [w225] -> w203
          tunnel: [w223] -> w202
          stop <- w224 stop-if-true
          w212 = u32 115200 items=["9600"=9600, "19200"=19200, "38400"=38400, "57600"=57600, "115200"=115200] ("Configure RS232 Baud Rate")
          n135 = Match Pattern(string=w220, regular expression="ASRL" ("format string")) -> (after substring=w213:string)  [unwired: 1 in, 3 out]
          n136 = Search/Split String(string=w213, search string/char (-)="::", offset (0)=1) -> (substring before match=w216:string)  [unwired: 2 out]
          n137 = Concatenate Strings("COM" ("string"), w216) -> (w217:string)
          n138 = call "Initialize.vi"("Configure RS232 Baud Rate"=w212, "error in (no error)"=w228, "Clear Error(True)"=TRUE, "ID Query (True)"=TRUE, "VISA resource name"=w217) -> ("error out"=w226:errorcluster, "VISA resource name out"=w211:refnum<visa-resource-name>)  [unwired: 3 in, 2 out]
          n139 = property on="Hillppot Comport" class="VISAName"("Value"=w211) -> ()  [unwired: 2 in, 2 out]
          n140 = call "Close.vi"("error in (no error)"=w226, "VISA resource name"=w211) -> ("error out"=w225:errorcluster)  [unwired: 9 in]
          n141 = Unbundle(w226) -> ("status"=w227:bool)  [unwired: 2 out]
          n142 = Not Equal?(x=w211, y=refnum<visa-resource-name> refnum) -> (x != y?=w222:bool)
          n143 = Not(x=w227) -> (.not. x?=w224:bool)
          n144 = And(x=w222, y=w224) -> (x .and. y?=w223:bool)
        }
        n145 = And(x=w201, y=w202) -> (x .and. y?=w200:bool)
        n146 = case shown="False" w200 {
          tunnel: [developer_test_sequence."Exit" ("Enum") developer_test_sequence."Idle State" ("Enum")] -> w208
          tunnel: w203 -> [_ w248]
          tunnel: [w245 w249] -> w207
          frame False {
            n147 = local write "status_bri"("Exit" ("status_bri")) -> ()
            n148 = call "MSG display box two buttons.vi"("input string"="Device are not connected") -> ("error out"=w245:errorcluster)  [unwired: 9 in, 1 out]
          }
          frame True {
            n149 = local write "status_bri"("Idle State" ("status_bri")) -> ()
            n150 = call "Main_Vi.vi"("error in (no error)"=w248, "State"="Init", "resource string"="USB0::0x2A8D::0x5001::MY58039196::INSTR") -> ("error out"=w249:errorcluster)  [unwired: 7 in, 1 out]
          }
        }
        n151 = call-poly "Enqueue Message.vi"("error in (no error)"=w207, "test sequence"=w208, "Message Queue"=w209) -> ("error out"=w210:errorcluster)  [unwired: 7 in, 1 out]
      }
      frame "Idle State" {
        n152 = property on="Start" class="Bool"("Visible"=TRUE) -> ()  [unwired: 2 in, 2 out]
        n153 = property on="Stop" class="Bool"("Visible"=FALSE) -> ()  [unwired: 2 in, 2 out]
        n154 = local write "status_bri"("Idle State" ("status_bri")) -> ()
      }
      frame "Start Display Board Auto Testing" {
        n155 = local write "status_bri"("Scan Barcode" ("status_bri")) -> ()
        n156 = call-poly "Enqueue Message.vi"("error in (no error)"=w260, "test sequence"=developer_test_sequence."Scan Barcode", "Message Queue"=w262) -> ("error out"=w261:errorcluster)  [unwired: 7 in, 1 out]
      }
      frame "Scan Barcode" {
        n157 = local read "Result indicators"() -> (w271:refnum<vi>[])
        n158 = call "Reset_resultbackground.vi"("error in (no error)"=w270, "appended array"=w271) -> ("error out"=w263:errorcluster)  [unwired: 9 in]
        n159 = call "DAQ_sub_DI-DO_.vi"("error in"=w263, "All OFF"=TRUE) -> ("error out"=w269:errorcluster)  [unwired: 8 in, 1 out]
        n160 = call "Read_Data.vi"("error in"=w263) -> ("string array"=w268:string[])  [unwired: 9 in, 1 out]
        n161 = property on="Limits" class="Arr (strict)"("Value"=w268) -> ()  [unwired: 2 in, 2 out]
        n162 = flat-sequence {
          tunnel: [w276] -> w265
          tunnel: [w275] -> w264
          tunnel: w269 -> [w283]
          tunnel: "1)Place the Battery\n\t2)Push theBattery. Make sure that it is locked\n\t3)Connect the Connectors\n\t4)Connect the Current probes\n\t5)Do DOWN the toggle" -> [w282]
          tunnel: [w281] -> w266
          tunnel: w265 -> [w280]
          tunnel: w264 -> [w279]
          frame #0 {
            n163 = call "Barcode user prompt.vi"() -> ("Module Type 2"=→"Module Type A/B":string, "BARCODE"=w275:string)  [unwired: 10 in]
            n164 = Equal?(x=w275, y="idel" ("before match")) -> (x = y?=w276:bool)
          }
          frame #1 {
            n165 = case shown="False" w280 {
              tunnel: w283 -> [w288 _]
              tunnel: w282 -> [w287 _]
              tunnel: [developer_test_sequence."Current contactor check" ("test sequence") developer_test_sequence."Idle State" ("test sequence")] -> w281
              tunnel: w279 -> [w285 _]
              frame False {
                n166 = local write "status_bri"("Checking Temp at Thermistor 1" ("status_bri")) -> ()
                n167 = local write "Array"(dbl[] [] ("Array")) -> ()
                n168 = call "MSG display box_2.vi"("1st Button"="Enter", "error in"=w288, "input string"=w287) -> ()  [unwired: 6 in, 3 out]
                n169 = invoke on="Temp value" class="Arr (strict)" method="Reinit To Default"() -> ()  [unwired: 3 in, 3 out]
                n170 = invoke on="Voltage health check" class="Arr (strict)" method="Reinit To Default"() -> ()  [unwired: 3 in, 3 out]
                n171 = invoke on="weld res" class="Arr (strict)" method="Reinit To Default"() -> ()  [unwired: 3 in, 3 out]
                n172 = invoke on="weld voltage" class="Arr (strict)" method="Reinit To Default"() -> ()  [unwired: 3 in, 3 out]
                "Module ID" <- w285
              }
              frame True {
              }
            }
          }
        }
        n173 = call-poly "Enqueue Message.vi"("error in (no error)"=w270, "test sequence"=w266, "Message Queue"=w274) -> ("error out"=w273:errorcluster)  [unwired: 7 in, 1 out]
      }
      frame "Current contactor check" {
        n174 = call "DAQ_sub_DI-DO_.vi"("error in"=w305, "All OFF"=TRUE) -> ("error out"=w303:errorcluster)  [unwired: 8 in, 1 out]
        n175 = local write "Update timer"(TRUE ("Update timer")) -> ()
        n176 = call "Main_Vi.vi"("ChannelList"="119", "error in (no error)"=w303, "Selection of reading"="Weld Resistance", "State"="Read") -> ("error out"=w300:errorcluster, "Val"=w302:dbl[])  [unwired: 6 in]
        n177 = local write "reset timer"(TRUE ("Update timer")) -> ()
        n178 = Index Array(array=w302, index=0) -> (element=w295:dbl)
        n179 = Multiply(x=1000.0, y=w295) -> (x*y=w294:dbl)
        n180 = Less?(x=w294, y=1.0) -> (x < y?=w297:bool)
        n181 = case shown="False" w297 {
          tunnel: [developer_test_sequence."Stop Display Board Auto Testing" ("test sequence") developer_test_sequence."Checking TEMP at Thermistor 1" ("test sequence")] -> w298
          frame False {
            n182 = call "MSG display box_2.vi"("Enable"=TRUE, "input string"="Check the load contactor ") -> ()  [unwired: 7 in, 3 out]
          }
          frame True {
          }
        }
        n183 = call-poly "Enqueue Message.vi"("error in (no error)"=w300, "test sequence"=w298, "Message Queue"=w309) -> ("error out"=w310:errorcluster)  [unwired: 7 in, 1 out]
      }
      frame "Checking TEMP at Thermistor 1" {
        w340 = TRUE ("ON/OFF")
        n184 = local write "Unlock"(FALSE ("Unlock")) -> ()
        n185 = property on="Stop" class="Bool"("Visible"=TRUE) -> ()  [unwired: 2 in, 2 out]
        n186 = property on="Start" class="Bool"("Visible"=FALSE) -> ()  [unwired: 2 in, 2 out]
        n187 = call "DAQ_sub_DI-DO_.vi"("error in"=w323, "ON/OFF"=w340, "Channel"=4) -> ("error out"=w343:errorcluster)  [unwired: 7 in, 1 out]
        n188 = call "DAQ_sub_DI-DO_.vi"("error in"=w343, "ON/OFF"=w340, "Channel"=5) -> ("error out"=w339:errorcluster)  [unwired: 7 in, 1 out]
        n189 = Get Date/Time In Seconds() -> (seconds since 1Jan1904=w320:timestamp)
        n190 = Get Date/Time String(seconds (now)=w320) -> (time string=→"Test Start Time":string)  [unwired: 2 in, 1 out]
        n191 = call "Main_Vi.vi"("ChannelList"="109", "error in (no error)"=w339, "Selection of reading"="Temperature", "State"="Read") -> ("error out"=w324:errorcluster, "Val"=w338:dbl[])  [unwired: 6 in]
        n192 = Index Array(array=w338, index=0) -> (element=w318:dbl)
        n193 = property on="Tempertaure Sensor" class="Str"() -> ("Value"=w317:string)  [unwired: 2 in, 2 out]
        n194 = call "Temperature_Calculation.vi"("R"=w318, "temp selection"=w317) -> ("temp"=w328:dbl)  [unwired: 9 in]
        n195 = property on="Output values" class="Clust (strict)"() -> ("Value"=w316:T1)  [unwired: 2 in, 2 out]
        n196 = call "DAQ_sub_DI-DO_.vi"("error in"=w324, "All OFF"=TRUE) -> ("error out"=w333:errorcluster)  [unwired: 8 in, 1 out]
        n197 = Unbundle By Name(w316) -> ("Temp-1"=w315:bool)
        n198 = local write "status_bri"("Checking Temp at Thermistor 2" ("status_bri")) -> ()
        n199 = case shown="True" w315 {
          tunnel: ["N/A" ("output string") w350] -> w336
          tunnel: w328 -> [_ w348]
          frame False {
          }
          frame True {
            n200 = Format Value(format string="%0.2f", value (0)=w348) -> (output string=w350:string)  [unwired: 1 in]
            n201 = local read "Array"() -> (w346:dbl[])
            n202 = Insert Into Array(array=w346, index=0, new element=w348) -> (w347:dbl[])
            n203 = local write "Array"(w347) -> ()
          }
        }
        "Thermistor 1" <- w336
        n204 = call-poly "Enqueue Message.vi"("error in (no error)"=w333, "test sequence"=developer_test_sequence."Checking TEMP at Thermistor 2", "Message Queue"=w334) -> ("error out"=w332:errorcluster)  [unwired: 7 in, 1 out]
      }
      frame "Checking TEMP at Thermistor 2" {
        w370 = TRUE ("ON/OFF")
        # "on 2,3 relays for mesure Temp-2"
        # "All off"
        n205 = call "DAQ_sub_DI-DO_.vi"("error in"=w373, "ON/OFF"=w370, "Channel"=2) -> ("error out"=w374:errorcluster)  [unwired: 7 in, 1 out]
        n206 = call "DAQ_sub_DI-DO_.vi"("error in"=w374, "ON/OFF"=w370, "Channel"=3) -> ("error out"=w369:errorcluster)  [unwired: 7 in, 1 out]
        n207 = call "Main_Vi.vi"("ChannelList"="109", "error in (no error)"=w369, "Selection of reading"="Temperature", "State"="Read") -> ("error out"=w354:errorcluster, "Val"=w368:dbl[])  [unwired: 6 in]
        n208 = local write "status_bri"("Checking Temp at Thermistor 3" ("status_bri")) -> ()
        n209 = property on="Tempertaure Sensor" class="Str"() -> ("Value"=w353:string)  [unwired: 2 in, 2 out]
        n210 = Index Array(array=w368, index=0) -> (element=w357:dbl)
        n211 = property on="Output values" class="Clust (strict)"() -> ("Value"=w352:T1)  [unwired: 2 in, 2 out]
        n212 = call "Temperature_Calculation.vi"("R"=w357, "temp selection"=w353) -> ("temp"=w358:dbl)  [unwired: 9 in]
        n213 = Unbundle By Name(w352) -> ("Temp-2"=w351:bool)
        n214 = case shown="True" w351 {
          tunnel: ["N/A" ("output string") w381] -> w366
          tunnel: w358 -> [_ w379]
          frame False {
          }
          frame True {
            n215 = local read "Array"() -> (w377:dbl[])
            n216 = Array Size(array=w377) -> (size(s)=w376:i32)
            n217 = Format Value(format string="%0.2f", value (0)=w379) -> (output string=w381:string)  [unwired: 1 in]
            n218 = Insert Into Array(array=w377, index=w376, new element=w379) -> (w378:dbl[])
            n219 = local write "Array"(w378) -> ()
          }
        }
        "Thermistor 2" <- w366
        n220 = call "DAQ_sub_DI-DO_.vi"("error in"=w354, "All OFF"=TRUE) -> ("error out"=w363:errorcluster)  [unwired: 8 in, 1 out]
        n221 = call-poly "Enqueue Message.vi"("error in (no error)"=w363, "test sequence"=developer_test_sequence."Checking TEMP at Thermistor 3", "Message Queue"=w365) -> ("error out"=w362:errorcluster)  [unwired: 7 in, 1 out]
      }
      frame "Checking TEMP at Thermistor 3" {
        w403 = TRUE ("ON/OFF")
        n222 = call "DAQ_sub_DI-DO_.vi"("error in"=w404, "ON/OFF"=w403, "Channel"=0) -> ("error out"=w405:errorcluster)  [unwired: 7 in, 1 out]
        n223 = call "DAQ_sub_DI-DO_.vi"("error in"=w405, "ON/OFF"=w403, "Channel"=1) -> ("error out"=w402:errorcluster)  [unwired: 7 in, 1 out]
        n224 = call "Main_Vi.vi"("ChannelList"="109", "error in (no error)"=w402, "Selection of reading"="Temperature", "State"="Read") -> ("error out"=w388:errorcluster, "Val"=w401:dbl[])  [unwired: 6 in]
        n225 = property on="Tempertaure Sensor" class="Str"() -> ("Value"=w384:string)  [unwired: 2 in, 2 out]
        n226 = Index Array(array=w401, index=0) -> (element=w391:dbl)
        n227 = property on="Output values" class="Clust (strict)"() -> ("Value"=w383:T1)  [unwired: 2 in, 2 out]
        n228 = call "Temperature_Calculation.vi"("R"=w391, "temp selection"=w384) -> ("temp"=w390:dbl)  [unwired: 9 in]
        n229 = call "DAQ_sub_DI-DO_.vi"("error in"=w388, "All OFF"=TRUE) -> ("error out"=w397:errorcluster)  [unwired: 8 in, 1 out]
        n230 = Unbundle By Name(w383) -> ("Temp-3"=w382:bool)
        n231 = case shown="True" w382 {
          tunnel: ["N/A" ("output string") w412] -> w399
          tunnel: w390 -> [_ w410]
          frame False {
          }
          frame True {
            n232 = local read "Array"() -> (w408:dbl[])
            n233 = Array Size(array=w408) -> (size(s)=w407:i32)
            n234 = Format Value(format string="%0.2f", value (0)=w410) -> (output string=w412:string)  [unwired: 1 in]
            n235 = Insert Into Array(array=w408, index=w407, new element=w410) -> (w409:dbl[])
            n236 = local write "Array"(w409) -> ()
          }
        }
        "Thermistor 3" <- w399
        n237 = local write "status_bri"("Checking Temp at Thermistor 4 (Ambient)" ("status_bri")) -> ()
        n238 = call-poly "Enqueue Message.vi"("error in (no error)"=w397, "test sequence"=developer_test_sequence."Checking TEMP at Thermistor 4 (Ambient)", "Message Queue"=w396) -> ("error out"=w398:errorcluster)  [unwired: 7 in, 1 out]
      }
      frame "Checking TEMP at Thermistor 4 (Ambient)" {
        # "If alll are uncheck (temp sensor)\nall will be N /A and BG as white"
        n239 = property on="Tempertaure Sensor" class="Str"() -> ("Value"=w436:string)  [unwired: 2 in, 2 out]
        n240 = call "Main_Vi.vi"("ChannelList"="120", "error in (no error)"=w472, "Selection of reading"="Temperature", "State"="Read") -> ("error out"=w465:errorcluster, "Val"=w474:dbl[])  [unwired: 6 in]
        n241 = local read "Limits"() -> (w446:string[])
        n242 = call <vilib>:"Application Directory.vi"() -> ("Application Directory"=w433:path)
        n243 = property on="Varaint Selection" class="Str"() -> ("Value"=w413:string)  [unwired: 2 in, 2 out]
        n244 = Index Array(array=w474, index=0) -> (element=w455:dbl)
        n245 = local read "Array"() -> (w442:dbl[])
        n246 = call "Limit.vi"("string array"=w446, "Enum"=T10."Temp") -> ("Limits"=w443:dbl[])  [unwired: 8 in, 1 out]
        n247 = call "Temperature_Calculation.vi"("R"=w455, "temp selection"=w436) -> ("temp"=w444:dbl)  [unwired: 9 in]
        n248 = Build Path(base path=w433, name or relative path=path "Data/Variant_details.ini") -> (appended path=w431:path)
        n249 = call "write_to_ini.vi"("Enum"=enum16{"Write", "Read variants", "Read Values"}."Read Values", "String"=w413, "configuration file path"=w431) -> ("Output values"=w434:T1)  [unwired: 5 in, 3 out]
        n250 = call "temp comprasion.vi"("Upper Limit"=w443, "Array"=w442, "Ambient temp"=w444) -> ("output array"=w439:bool[], "pass or fail"=w441:T13, "temp array"=→"Temp value":dbl[])  [unwired: 6 in]
        n251 = Unbundle By Name(w434) -> ("Temp-1"=w418:bool, "Temp-2"=w417:bool, "Temp-3"=w416:bool)
        n252 = Format Value(format string="%0.2f", value (0)=w444) -> (output string=→"Thermistor 4 (Ambient)":string)  [unwired: 1 in]
        n253 = Index Array(array=w441, index=0) -> (element=w425:T14)
        n254 = Index Array(array=w441, index=1) -> (element=w423:T14)
        n255 = Index Array(array=w441, index=2) -> (element=w421:T14)
        n256 = Index Array(array=w441, index=3) -> (element=w419:T14)
        n257 = call "Final_result.vi"("Boolean array"=w439) -> ("Status Color"=w427:u32, "Status"=w429:string)  [unwired: 8 in, 1 out]
        n258 = Build Array(w418, w417, w416) -> (w415:bool[])
        n259 = Or Array Elements(Boolean array=w415) -> (logical OR=w414:bool)
        n260 = case shown="False" w414 {
          tunnel: ["N/A" ("Status") w483] -> w430
          tunnel: w429 -> [_ w483]
          tunnel: [u32 16448250 ("Status Color") w482] -> w428
          tunnel: w427 -> [_ w482]
          tunnel: [w475 w481] -> w426
          tunnel: w425 -> [_ w481]
          tunnel: [w475 w480] -> w424
          tunnel: w423 -> [_ w480]
          tunnel: [w475 w479] -> w422
          tunnel: w421 -> [_ w479]
          tunnel: [w475 w478] -> w420
          tunnel: w419 -> [_ w478]
          frame False {
            w475 = T15 {"measured value"="N/A", "N/A", "Status Color"=16448250}
          }
          frame True {
          }
        }
        "final temp result" <- w430
        n261 = call-poly "Enqueue Message.vi"("error in (no error)"=w465, "test sequence"=developer_test_sequence."Voltage Health Check", "Message Queue"=w466) -> ("error out"=w467:errorcluster)  [unwired: 7 in, 1 out]
        n262 = local write "status_bri"("Voltage health Check" ("status_bri")) -> ()
        n263 = Unbundle(w420) -> ("measured value"=→"Ambient Temperature imbalance":string, →"Ambient Temperature imbalance Result":string, "Text.Text Colors:BG Color"=w451:u32)
        n264 = Unbundle(w422) -> ("measured value"=→"8S- temperaturen imbalance":string, →"8S- temperature imbalance Result":string, "Text.Text Colors:BG Color"=w452:u32)
        n265 = Unbundle(w424) -> ("measured value"=→"Min Temperature":string, →"Min Temperature Result":string, "Text.Text Colors:BG Color"=w453:u32)
        n266 = Unbundle(w426) -> ("measured value"=→"Max Temperature":string, →"Max Temperature Result":string, "Text.Text Colors:BG Color"=w454:u32)
        n267 = property on="final temp result" class="Str"("Text.BGColor"=w428) -> ()  [unwired: 2 in, 2 out]
        n268 = property on="Ambient Temperature imbalance Result" class="Str"("Text.BGColor"=w451) -> ()  [unwired: 2 in, 2 out]
        n269 = property on="8S- temperature imbalance Result" class="Str"("Text.BGColor"=w452) -> ()  [unwired: 2 in, 2 out]
        n270 = property on="Min Temperature Result" class="Str"("Text.BGColor"=w453) -> ()  [unwired: 2 in, 2 out]
        n271 = property on="Max Temperature Result" class="Str"("Text.BGColor"=w454) -> ()  [unwired: 2 in, 2 out]
      }
      frame "Voltage Health Check" {
        w515 = i16 4 ("precision (6)")
        n272 = local read "Module Type A/B"() -> (w561:string)
        n273 = call "Main_Vi.vi"("ChannelList"="101:108", "error in (no error)"=w597, "Selection of reading"="Cell Voltage", "State"="Read") -> ("error out"=w568:errorcluster, "Val"=w565:dbl[])  [unwired: 6 in]
        n274 = Array Subset(array=w565, index=0, length=8) -> (w562:dbl[])
        n275 = case shown="\"B\", Default" w561 {
          tunnel: w562 -> [w599 w601]
          tunnel: [w598 w602] -> w506
          frame "B", Default {
            n276 = Reverse 1D Array(array=w599) -> (reversed array=w598:dbl[])
          }
          frame "A" {
            n277 = Reverse 1D Array(array=w601) -> (reversed array=w600:dbl[])
            n278 = call "negative to postive.vi"("Array"=w600) -> ("Array 2"=w602:dbl[])  [unwired: 10 in]
          }
        }
        n279 = Add Array Elements(numeric array=w506) -> (sum=w500:dbl)
        n280 = Array Max & Min(array=w506) -> (max value=w535:dbl, min value=w534:dbl)  [unwired: 2 out]
        n281 = Subtract(x=w535, y=w534) -> (x-y=w487:dbl)
        n282 = Multiply(x=w487, y=1000.0) -> (x*y=w488:dbl)
        n283 = local read "Limits"() -> (w519:string[])
        n284 = Build Array(w535, w534, w500, w488) -> (w560:dbl[])
        n285 = call "Limit.vi"("string array"=w519, "Enum"=T10."Voltage") -> ("Limits"=w508:dbl[])  [unwired: 8 in, 1 out]
        n286 = Insert Into Array(array=w506, new element=w560) -> (w493:dbl[])  [unwired: 1 in]
        "Voltage health check" <- w493
        n287 = Index Array(array=w493, index=10) -> (element=w491:dbl)
        n288 = Array Subset(array=w493, index=0, length=10) -> (w505:dbl[])
        n289 = Index Array(array=w493, index=11) -> (element=w489:dbl)
        n290 = Index Array(array=w508, index=11) -> (element=w501:dbl)
        n291 = call "verify_results_array.vi"("precision (6)"=w515, "Mesured values"=w505, "Lower Limit"=w508, "comparison"=comparison_selection."greater than?") -> ("Pass or fail array"=w512:bool[], "Array"=w514:T13)  [unwired: 5 in, 1 out]
        n292 = Build Array(w491) -> (w490:dbl[])
        n293 = Build Array(w489) -> (w517:dbl[])
        n294 = Build Array(w501) -> (w507:dbl[])
        n295 = call "verify_results_array.vi"("Mesured values"=w490, "Lower Limit"=dbl[] [23.5], "Upper Limit"=dbl[] [28.5], "comparison"=comparison_selection."in-range?") -> ("Pass or fail array"=w494:bool[], "Array"=w495:T13)  [unwired: 5 in, 1 out]
        n296 = call "verify_results_array.vi"("precision (6)"=w515, "Mesured values"=w517, "Upper Limit"=w507, "comparison"=comparison_selection."less than?") -> ("Pass or fail array"=w511:bool[], "Array"=w496:T13)  [unwired: 5 in, 1 out]
        n297 = Insert Into Array(array=w514, new element #1=w495, new element #2=w496) -> (w513:T13)  [unwired: 1 in]
        n298 = Insert Into Array(array=w512, new element #1=w511, new element #2=w494) -> (w510:bool[])  [unwired: 1 in]
        n299 = Index Array(array=w513, index=9) -> (element=w557:T14)
        n300 = Index Array(array=w513, index=0) -> (element=w593:T14)
        n301 = Index Array(array=w513, index=1) -> (element=w592:T14)
        n302 = Index Array(array=w513, index=2) -> (element=w591:T14)
        n303 = Index Array(array=w513, index=3) -> (element=w590:T14)
        n304 = Index Array(array=w513, index=4) -> (element=w589:T14)
        n305 = Index Array(array=w513, index=5) -> (element=w588:T14)
        n306 = Index Array(array=w513, index=6) -> (element=w587:T14)
        n307 = Index Array(array=w513, index=7) -> (element=w586:T14)
        n308 = Index Array(array=w513, index=8) -> (element=w559:T14)
        n309 = Unbundle(w557) -> ("measured value"=→"Min voltage":string, →"Min voltage Result":string, "Text.Text Colors:BG Color"=w524:u32)
        n310 = Unbundle(w593) -> ("measured value"=→"Cell 1":string, →"Cell 1 Result":string, "Text.Text Colors:BG Color"=w533:u32)
        n311 = Unbundle(w592) -> ("measured value"=→"Cell 2":string, →"Cell 2 Result":string, "Text.Text Colors:BG Color"=w532:u32)
        n312 = Unbundle(w591) -> ("measured value"=→"Cell 3":string, →"Cell 3 Result":string, "Text.Text Colors:BG Color"=w531:u32)
        n313 = Unbundle(w590) -> ("measured value"=→"Cell 4":string, →"Cell 4 Result":string, "Text.Text Colors:BG Color"=w530:u32)
        n314 = Unbundle(w586) -> ("measured value"=→"Cell 8":string, →"Cell 8 Result":string, "Text.Text Colors:BG Color"=w526:u32)
        n315 = Unbundle(w588) -> ("measured value"=→"Cell 6":string, →"Cell 6 Result":string, "Text.Text Colors:BG Color"=w527:u32)
        n316 = Unbundle(w587) -> ("measured value"=→"Cell 7":string, →"Cell 7 Result":string, "Text.Text Colors:BG Color"=w529:u32)
        n317 = Unbundle(w589) -> ("measured value"=→"Cell 5":string, →"Cell 5 Result":string, "Text.Text Colors:BG Color"=w528:u32)
        n318 = Unbundle(w559) -> ("measured value"=→"Max Voltage":string, →"Max Voltage Result":string, "Text.Text Colors:BG Color"=w525:u32)
        n319 = property on="Min voltage Result" class="Str"("Text.BGColor"=w524) -> ()  [unwired: 2 in, 2 out]
        n320 = property on="Max Voltage Result" class="Str"("Text.BGColor"=w525) -> ()  [unwired: 2 in, 2 out]
        n321 = property on="Cell 4 Result" class="Str"("Text.BGColor"=w530) -> ()  [unwired: 2 in, 2 out]
        n322 = property on="Cell 3 Result" class="Str"("Text.BGColor"=w531) -> ()  [unwired: 2 in, 2 out]
        n323 = property on="Cell 6 Result" class="Str"("Text.BGColor"=w527) -> ()  [unwired: 2 in, 2 out]
        n324 = property on="Cell 7 Result" class="Str"("Text.BGColor"=w529) -> ()  [unwired: 2 in, 2 out]
        n325 = property on="Cell 8 Result" class="Str"("Text.BGColor"=w526) -> ()  [unwired: 2 in, 2 out]
        n326 = property on="Cell 2 Result" class="Str"("Text.BGColor"=w532) -> ()  [unwired: 2 in, 2 out]
        n327 = property on="Cell 5 Result" class="Str"("Text.BGColor"=w528) -> ()  [unwired: 2 in, 2 out]
        n328 = property on="Cell 1 Result" class="Str"("Text.BGColor"=w533) -> ()  [unwired: 2 in, 2 out]
        n329 = call "Final_result.vi"("Boolean array"=w510) -> ("Status Color"=w520:u32, "Status"=→"Final Voltage test result":string)  [unwired: 8 in, 1 out]
        n330 = Index Array(array=w513, index=10) -> (element=w556:T14)
        n331 = Index Array(array=w513, index=11) -> (element=w554:T14)
        n332 = Unbundle(w556) -> ("measured value"=→"8S - Voltage":string, →"8S - Voltage Result":string, "Text.Text Colors:BG Color"=w523:u32)
        n333 = Unbundle(w554) -> ("measured value"=→"Cell 8S - Voltage Imbalance (mv)":string, →"Cell 8S - Voltage Imbalance (mv) Result":string, "Text.Text Colors:BG Color"=w522:u32)
        n334 = property on="Final Voltage test result" class="Str"("Text.BGColor"=w520) -> ()  [unwired: 2 in, 2 out]
        n335 = property on="8S - Voltage Result" class="Str"("Text.BGColor"=w523) -> ()  [unwired: 2 in, 2 out]
        n336 = property on="Cell 8S - Voltage Imbalance (mv) Result" class="Str"("Text.BGColor"=w522) -> ()  [unwired: 2 in, 2 out]
        n337 = call-poly "Enqueue Message.vi"("error in (no error)"=w568, "test sequence"=developer_test_sequence."Hillpot connector check", "Message Queue"=w567) -> ("error out"=w569:errorcluster)  [unwired: 7 in, 1 out]
        n338 = local write "status_bri"("Hipot Connector Check" ("status_bri")) -> ()
      }
      frame "Hillpot connector check" {
        w620 = TRUE ("ON/OFF")
        n339 = local read "Limits"() -> (w608:string[])
        n340 = call "DAQ_sub_DI-DO_.vi"("error in"=w619, "ON/OFF"=w620, "Channel"=7) -> ("error out"=w623:errorcluster)  [unwired: 7 in, 1 out]
        n341 = Index Array(array=w608, index=18) -> (element=w607:string)
        n342 = call "mSec wait.vi"("Error in"=w623, "mSec wait"=u32 500) -> ("Error out"=w612:errorcluster)  [unwired: 9 in]
        n343 = property on="Hillppot Comport" class="VISAName"() -> ("Value"=w603:refnum<visa-resource-name>)  [unwired: 2 in, 2 out]
        n344 = Decimal String To Number(string=w607) -> (number=w606:i32)  [unwired: 2 in, 1 out]
        n345 = call "DAQ_sub_DI-DO_.vi"("error in"=w612, "ON/OFF"=w620, "Channel"=8) -> ("error out"=w618:errorcluster)  [unwired: 7 in, 1 out]
        n346 = call "HIPOT-GPT9803 IR TEST.vi"("error in"=w618, "IR LO SET resistance value(M£[)"=w606, "VISA resource name"=w603) -> ("error out"=w614:errorcluster, "RESULT"=w609:bool)  [unwired: 5 in, 2 out]
        n347 = Not(x=w609) -> (.not. x?=w604:bool)
        n348 = case shown="True" w604 {
          tunnel: [developer_test_sequence."Stop Display Board Auto Testing" ("test sequence") developer_test_sequence."INSULATION Resistance test (Baseplate to Negative)" ("test sequence")] -> w617
          frame False {
            n349 = local write "status_bri"("Report" ("status_bri")) -> ()
            n350 = call "MSG display box_2.vi"("Enable"=TRUE, "input string"="Check the Contact for Base plate") -> ()  [unwired: 7 in, 3 out]
          }
          frame True {
            n351 = local write "status_bri"("INSULATION Resistance test (Baseplate to Negative)" ("status_bri")) -> ()
          }
        }
        n352 = call "DAQ_sub_DI-DO_.vi"("error in"=w614, "All OFF"=TRUE) -> ("error out"=w610:errorcluster)  [unwired: 8 in, 1 out]
        n353 = call-poly "Enqueue Message.vi"("error in (no error)"=w610, "test sequence"=w617, "Message Queue"=w616) -> ("error out"=w615:errorcluster)  [unwired: 7 in, 1 out]
      }
      frame "INSULATION Resistance test (Baseplate to Negative)" {
        w657 = TRUE ("ON/OFF")
        n354 = local read "Limits"() -> (w639:string[])
        n355 = call "DAQ_sub_DI-DO_.vi"("error in"=w656, "ON/OFF"=w657, "Channel"=8) -> ("error out"=w660:errorcluster)  [unwired: 7 in, 1 out]
        n356 = Index Array(array=w639, index=18) -> (element=w638:string)
        n357 = call "mSec wait.vi"("Error in"=w660, "mSec wait"=u32 500) -> ("Error out"=w646:errorcluster)  [unwired: 9 in]
        n358 = property on="Hillppot Comport" class="VISAName"() -> ("Value"=w630:refnum<visa-resource-name>)  [unwired: 2 in, 2 out]
        n359 = Decimal String To Number(string=w638) -> (number=w637:i32)  [unwired: 2 in, 1 out]
        n360 = call "DAQ_sub_DI-DO_.vi"("error in"=w646, "ON/OFF"=w657, "Channel"=9) -> ("error out"=w655:errorcluster)  [unwired: 7 in, 1 out]
        n361 = call "HIPOT-GPT9803 IR TEST.vi"("error in"=w655, "IR LO SET resistance value(M£[)"=w637, "VISA resource name"=w630) -> ("error out"=w648:errorcluster, "Impedance"=w634:string, "RESULT"=w641:bool)  [unwired: 5 in, 1 out]
        n362 = case shown="False" w641 {
          tunnel: [developer_test_sequence."Stop Display Board Auto Testing" ("test sequence") developer_test_sequence."INSULATION Resistance test (Baseplate to Positive)" ("test sequence")] -> w651
          frame False {
            n363 = local write "status_bri"("Report" ("status_bri")) -> ()
            n364 = property on="Final Insulation Resistance Result" class="Str"("Text.BGColor"=u32 16711680 ("Text.Text Colors:BG Color")) -> ()  [unwired: 2 in, 2 out]
            n365 = property on="Final Insulation Resistance Result" class="Str"("Value"="FAIL" ("Final Insulation Resistance Result")) -> ()  [unwired: 2 in, 2 out]
          }
          frame True {
            n366 = local write "status_bri"("INSULATION Resistance test (Baseplate to Positive)" ("status_bri")) -> ()
          }
        }
        n367 = Select(t=u32 6618880 ("Text.Text Colors:BG Color"), s=w641, f=u32 16711680 ("Text.Text Colors:BG Color")) -> (s? t:f=w642:u32)
        n368 = Search/Split String(string=w634, search string/char (-)="M") -> (substring before match=w633:string)  [unwired: 1 in, 2 out]
        n369 = Select(t="PASS", s=w641, f="FAIL") -> (s? t:f=→"Baseplate to Negative Result":string)
        n370 = property on="Baseplate to Negative Result" class="Str"("Text.BGColor"=w642) -> ()  [unwired: 2 in, 2 out]
        n371 = Decimal String To Number(string=w633) -> (number=w632:i32)  [unwired: 2 in, 1 out]
        n372 = Number To Decimal String(number=w632) -> (decimal integer string=→"Baseplate to Negative":string)  [unwired: 1 in]
        n373 = call "DAQ_sub_DI-DO_.vi"("error in"=w648, "All OFF"=TRUE) -> ("error out"=w644:errorcluster)  [unwired: 8 in, 1 out]
        n374 = call-poly "Enqueue Message.vi"("error in (no error)"=w644, "test sequence"=w651, "Message Queue"=w650) -> ("error out"=w649:errorcluster)  [unwired: 7 in, 1 out]
      }
      frame "INSULATION Resistance test (Baseplate to Positive)" {
        w697 = TRUE ("ON/OFF")
        n375 = call "mSec wait.vi"("Error in"=w696, "mSec wait"=u32 2000) -> ("Error out"=w688:errorcluster)  [unwired: 9 in]
        n376 = local read "Limits"() -> (w676:string[])
        n377 = call "DAQ_sub_DI-DO_.vi"("error in"=w688, "ON/OFF"=w697, "Channel"=6) -> ("error out"=w700:errorcluster)  [unwired: 7 in, 1 out]
        n378 = Index Array(array=w676, index=18) -> (element=w674:string)
        n379 = call "mSec wait.vi"("Error in"=w700, "mSec wait"=u32 500) -> ("Error out"=w684:errorcluster)  [unwired: 9 in]
        n380 = property on="Hillppot Comport" class="VISAName"() -> ("Value"=w667:refnum<visa-resource-name>)  [unwired: 2 in, 2 out]
        n381 = Decimal String To Number(string=w674) -> (number=w673:i32)  [unwired: 2 in, 1 out]
        n382 = call "DAQ_sub_DI-DO_.vi"("error in"=w684, "ON/OFF"=w697, "Channel"=7) -> ("error out"=w695:errorcluster)  [unwired: 7 in, 1 out]
        n383 = call "HIPOT-GPT9803 IR TEST.vi"("error in"=w695, "IR LO SET resistance value(M£[)"=w673, "VISA resource name"=w667) -> ("error out"=w686:errorcluster, "Impedance"=w671:string, "RESULT"=w680:bool)  [unwired: 5 in, 1 out]
        n384 = case shown="True" w680 {
          tunnel: [developer_test_sequence."Stop Display Board Auto Testing" ("test sequence") developer_test_sequence."WELD Resistance Test" ("test sequence")] -> w689
          frame False {
            n385 = local write "status_bri"("Report" ("status_bri")) -> ()
          }
          frame True {
            n386 = local write "status_bri"("WELD Resistance Test" ("status_bri")) -> ()
          }
        }
        n387 = Select(t=u32 6618880 ("Text.Text Colors:BG Color"), s=w680, f=u32 16711680 ("Text.Text Colors:BG Color")) -> (s? t:f=w679:u32)
        n388 = call "DAQ_sub_DI-DO_.vi"("error in"=w686, "All OFF"=TRUE) -> ("error out"=w690:errorcluster)  [unwired: 8 in, 1 out]
        n389 = property on="Baseplate to Positive Result" class="Str"("Text.BGColor"=w679) -> ()  [unwired: 2 in, 2 out]
        n390 = Search/Split String(string=w671, search string/char (-)="M") -> (substring before match=w670:string)  [unwired: 1 in, 2 out]
        n391 = Select(t="PASS", s=w680, f="FAIL") -> (s? t:f=→"Baseplate to Positive Result":string)
        n392 = Decimal String To Number(string=w670) -> (number=w669:i32)  [unwired: 2 in, 1 out]
        n393 = Number To Decimal String(number=w669) -> (decimal integer string=→"Baseplate to Positive":string)  [unwired: 1 in]
        n394 = call-poly "Enqueue Message.vi"("error in (no error)"=w690, "test sequence"=w689, "Message Queue"=w691) -> ("error out"=w678:errorcluster)  [unwired: 7 in, 1 out]
        n395 = flat-sequence {
          tunnel: w678 -> [w708]
          tunnel: [w708] -> w677
          frame #0 {
            n396 = local read "Baseplate to Negative Result"() -> (w714:string)
            n397 = local read "Baseplate to Positive Result"() -> (w711:string)
            n398 = Equal?(x=w714, y="PASS") -> (x = y?=w710:bool)
            n399 = Equal?(x=w711, y="PASS") -> (x = y?=w709:bool)
            n400 = And(x=w710, y=w709) -> (x .and. y?=w703:bool)
            n401 = Select(t=u32 6618880 ("Text.Text Colors:BG Color"), s=w703, f=u32 16711680 ("Text.Text Colors:BG Color")) -> (s? t:f=w701:u32)
            n402 = Select(t="PASS", s=w703, f="FAIL") -> (s? t:f=→"Final Insulation Resistance Result":string)
            n403 = property on="Final Insulation Resistance Result" class="Str"("Text.BGColor"=w701) -> ()  [unwired: 2 in, 2 out]
          }
        }
      }
      frame "Voltage helath check before weld resistance" {
        # "Test Skipped"
        n404 = call "Main_Vi.vi"("ChannelList"="101:108", "error in (no error)"=w738, "Selection of reading"="Cell Voltage", "State"="Read") -> ("error out"=w733:errorcluster, "Val"=w731:dbl[])  [unwired: 6 in]
        n405 = local read "Module Type A/B"() -> (w727:string)
        n406 = Array Subset(array=w731, index=0, length=8) -> (w728:dbl[])
        n407 = case shown="\"A\"" w727 {
          tunnel: w728 -> [w741 w743]
          tunnel: [w741 w742] -> w719
          frame "B", Default {
          }
          frame "A" {
            n408 = call "negative to postive.vi"("Array"=w743) -> ("Array 2"=w742:dbl[])  [unwired: 10 in]
          }
        }
        n409 = local read "Limits"() -> (w726:string[])
        n410 = call "Limit.vi"("string array"=w726, "Enum"=T10."Voltage befor WR") -> ("Limits"=w725:dbl[])  [unwired: 8 in, 1 out]
        n411 = call "verify_results_array.vi"("Mesured values"=w719, "Lower Limit"=w725, "comparison"=comparison_selection."greater than?") -> ("Pass or fail array"=w724:bool[])  [unwired: 6 in, 2 out]
        n412 = call "Final_result.vi"("Boolean array"=w724) -> ("logical AND"=w723:bool)  [unwired: 8 in, 2 out]
        n413 = case shown="True" w723 {
          tunnel: [developer_test_sequence."Stop Display Board Auto Testing" ("test sequence") developer_test_sequence."WELD Resistance Test" ("test sequence")] -> w722
          frame False {
          }
          frame True {
          }
        }
        n414 = call-poly "Enqueue Message.vi"("error in (no error)"=w733, "test sequence"=w722, "Message Queue"=w732) -> ("error out"=w734:errorcluster)  [unwired: 7 in, 1 out]
      }
      frame "WELD Resistance Test" {
        n415 = call "DAQ_sub_DI-DO_.vi"("error in"=w791, "ON/OFF"=TRUE, "Channel"=10) -> ("error out"=w790:errorcluster)  [unwired: 7 in, 1 out]
        n416 = call "mSec wait.vi"("Error in"=w790, "mSec wait"=u32 1000) -> ("Error out"=w754:errorcluster)  [unwired: 9 in]
        n417 = flat-sequence {
          tunnel: [w842] -> w755
          tunnel: w754 -> [w842]
          tunnel: [w841] -> w750
          frame #0 {
            n418 = Tick Count (ms)() -> (millisecond timer value=w841:u32)
          }
        }
        n419 = call "Main_Vi.vi"("ChannelList"="119", "error in (no error)"=w755, "Selection of reading"="Weld Resistance", "State"="Read") -> ("error out"=w759:errorcluster, "Val"=w764:dbl[])  [unwired: 6 in]
        n420 = call "Main_Vi.vi"("ChannelList"="110:118", "error in (no error)"=w759, "Selection of reading"="Cell Voltage", "State"="Read") -> ("error out"=w752:errorcluster, "Val"=w783:dbl[])  [unwired: 6 in]
        n421 = Index Array(array=w764, index=0) -> (element=w770:dbl)
        n422 = flat-sequence {
          tunnel: [w840] -> w753
          tunnel: w752 -> [w840]
          tunnel: [w839] -> w751
          frame #0 {
            n423 = Tick Count (ms)() -> (millisecond timer value=w839:u32)
          }
        }
        n424 = Divide(x=w770, y=0.16666) -> (x/y=w747:dbl)
        n425 = Array Subset(array=w783, index=0, length=9) -> (w757:dbl[])
        n426 = local read "Limits"() -> (w772:string[])
        n427 = Reverse 1D Array(array=w757) -> (reversed array=w756:dbl[])
        "weld voltage" <- w756
        n428 = Multiply(x=1000.0, y=w747) -> (x*y=w758:dbl)
        "Current" <- w758
        n429 = call "Limit.vi"("string array"=w772, "Enum"=T10."Weld resistance") -> ("Limits 2"=w744:dbl[], "Limits"=w745:dbl[])  [unwired: 8 in]
        n430 = call "weld_resistance calculation.vi"("Numeric"=w758, "Val"=w756) -> ("Array 2"=w787:dbl[])  [unwired: 9 in]
        "weld res" <- w787
        n431 = Greater?(x=w758, y=40.0) -> (0:w768:bool)
        n432 = case shown="False" w768 {
          frame False {
            n433 = call "DAQ_sub_DI-DO_.vi"("All OFF"=TRUE) -> ()  [unwired: 9 in, 2 out]
            n434 = call "MSG display box_2.vi"("input string"="Check the contactor or MCB of the  Load Box") -> ()  [unwired: 8 in, 3 out]
          }
          frame True {
          }
        }
        n435 = Subtract(x=w751, y=w750) -> (x-y=→"m second":u32)
        n436 = call "verify_results_array.vi"("precision (6)"=i16 3, "Mesured values"=w787, "Lower Limit"=w744, "Upper Limit"=w745, "comparison"=comparison_selection."in-range?") -> ("Pass or fail array"=w782:bool[], "Array"=w776:T13)  [unwired: 4 in, 1 out]
        n437 = call "DAQ_sub_DI-DO_.vi"("error in"=w753, "ON/OFF"=FALSE, "Channel"=10) -> ("error out"=w763:errorcluster)  [unwired: 7 in, 1 out]
        n438 = Index Array(array=w776, index=8) -> (element=w826:T14)
        n439 = Index Array(array=w776, index=4) -> (element=w829:T14)
        n440 = Index Array(array=w776, index=5) -> (element=w828:T14)
        n441 = Index Array(array=w776, index=6) -> (element=w827:T14)
        n442 = Index Array(array=w776, index=7) -> (element=w777:T14)
        n443 = Index Array(array=w776, index=0) -> (element=w833:T14)
        n444 = Index Array(array=w776, index=1) -> (element=w832:T14)
        n445 = Index Array(array=w776, index=2) -> (element=w831:T14)
        n446 = Index Array(array=w776, index=3) -> (element=w830:T14)
        n447 = Unbundle(w827) -> ("measured value"=→"Cell 6 - Cell 7":string, →"Cell 6 - Cell 7 Result":string, "Text.Text Colors:BG Color"=w805:u32)
        n448 = Unbundle(w777) -> ("measured value"=→"Cell 7 - Cell 8":string, →"Cell 7 - Cell 8 Result":string, "Text.Text Colors:BG Color"=w773:u32)
        n449 = Unbundle(w826) -> ("measured value"=→"Cell 8 (End Busbar)":string, →"Cell 8 (End Busbar) Result":string, "Text.Text Colors:BG Color"=w804:u32)
        n450 = Unbundle(w833) -> ("measured value"=→"Cell 1 (End Blusbar)":string, →"Cell 1 (End Blusbar) Result":string, "Text.Text Colors:BG Color"=w807:u32)
        n451 = Unbundle(w832) -> ("measured value"=→"Cell 1 - Cell 2":string, →"Cell 1 - Cell 2 Result":string, "Text.Text Colors:BG Color"=w806:u32)
        n452 = Unbundle(w831) -> ("measured value"=→"Cell 2 - Cell 3":string, →"Cell 2 - Cell 3 Result":string, "Text.Text Colors:BG Color"=w797:u32)
        n453 = Unbundle(w830) -> ("measured value"=→"Cell 3 - Cell 4":string, →"Cell 3 - Cell 4 Result":string, "Text.Text Colors:BG Color"=w796:u32)
        n454 = Unbundle(w829) -> ("measured value"=→"Cell 4 -Cell 5":string, →"Cell 4 -Cell 5 Result":string, "Text.Text Colors:BG Color"=w794:u32)
        n455 = Unbundle(w828) -> ("measured value"=→"Cell 5 - Cell 6":string, →"Cell 5 - Cell 6 Result":string, "Text.Text Colors:BG Color"=w795:u32)
        n456 = property on="Cell 1 (End Blusbar) Result" class="Str"("Text.BGColor"=w807) -> ()  [unwired: 2 in, 2 out]
        n457 = property on="Cell 1 - Cell 2 Result" class="Str"("Text.BGColor"=w806) -> ()  [unwired: 2 in, 2 out]
        n458 = property on="Cell 2 - Cell 3 Result" class="Str"("Text.BGColor"=w797) -> ()  [unwired: 2 in, 2 out]
        n459 = property on="Cell 3 - Cell 4 Result" class="Str"("Text.BGColor"=w796) -> ()  [unwired: 2 in, 2 out]
        n460 = property on="Cell 4 -Cell 5 Result" class="Str"("Text.BGColor"=w794) -> ()  [unwired: 2 in, 2 out]
        n461 = property on="Cell 5 - Cell 6 Result" class="Str"("Text.BGColor"=w795) -> ()  [unwired: 2 in, 2 out]
        n462 = property on="Cell 6 - Cell 7 Result" class="Str"("Text.BGColor"=w805) -> ()  [unwired: 2 in, 2 out]
        n463 = property on="Cell 7 - Cell 8 Result" class="Str"("Text.BGColor"=w773) -> ()  [unwired: 2 in, 2 out]
        n464 = property on="Cell 8 (End Busbar) Result" class="Str"("Text.BGColor"=w804) -> ()  [unwired: 2 in, 2 out]
        n465 = call "Final_result.vi"("Boolean array"=w782) -> ("Status Color"=w766:u32, "Status"=→"Final Weld Resistance Result":string)  [unwired: 8 in, 1 out]
        n466 = property on="Final Weld Resistance Result" class="Str"("Text.BGColor"=w766) -> ()  [unwired: 2 in, 2 out]
        n467 = call-poly "Enqueue Message.vi"("error in (no error)"=w763, "test sequence"=developer_test_sequence."Stop Display Board Auto Testing", "Message Queue"=w835) -> ("error out"=w834:errorcluster)  [unwired: 7 in, 1 out]
      }
      frame "Stop Display Board Auto Testing" {
        n468 = call-poly "Enqueue Message.vi"("test sequence"=developer_test_sequence."All Pass", "Message Queue"=w846) -> ("error out"=w847:errorcluster)  [unwired: 8 in, 1 out]
      }
      frame "All Pass" {
        w861 = FALSE ("Update timer")
        # "If all are uncheck then dummy\npass for temp else it status"
        n469 = property on="Varaint Selection" class="Str"() -> ("Value"=w848:string)  [unwired: 2 in, 2 out]
        n470 = call <vilib>:"Application Directory.vi"() -> ("Application Directory"=w858:path)
        n471 = property on="Update timer" class="Bool (strict)"("Value"=w861) -> ()  [unwired: 2 in, 2 out]
        n472 = property on="reset timer" class="Bool (strict)"("Value"=w861) -> ()  [unwired: 2 in, 2 out]
        n473 = Build Path(base path=w858, name or relative path=path "Data/Variant_details.ini") -> (appended path=w856:path)
        n474 = call "write_to_ini.vi"("Enum"=enum16{"Write", "Read variants", "Read Values"}."Read Values", "String"=w848, "configuration file path"=w856) -> ("Output values"=w859:T1)  [unwired: 5 in, 3 out]
        n475 = Unbundle By Name(w859) -> ("Temp-1"=w855:bool, "Temp-2"=w854:bool, "Temp-3"=w853:bool)
        n476 = Build Array(w855, w854, w853) -> (w852:bool[])
        n477 = Or Array Elements(Boolean array=w852) -> (logical OR=w849:bool)
        n478 = case shown="True" w849 {
          tunnel: ["PASS" ("final temp result") w872] -> w850
          frame False {
          }
          frame True {
            n479 = local read "final temp result"() -> (w872:string)
          }
        }
        n480 = local read "Final Insulation Resistance Result"() -> (w866:string)
        n481 = local read "Final Weld Resistance Result"() -> (w851:string)
        n482 = local read "Final Voltage test result"() -> (w865:string)
        n483 = Build Array(w866, w865, w851, w850) -> (w864:string[])
        n484 = for {
          tunnel: w864 -> [w875] mode=indexing
          tunnel: [w873] -> w863 mode=indexing
          n485 = Equal?(x=w875, y="PASS") -> (x = y?=w873:bool)
        }
        n486 = And Array Elements(Boolean array=w863) -> (logical AND=w862:bool)
        "Result" <- w862
        n487 = call "PASS_FAIL_Prompt.vi"("Result"=w862) -> ()  [unwired: 11 in]
        n488 = call-poly "Enqueue Message.vi"("error in (no error)"=w867, "test sequence"=developer_test_sequence."Report" ("Enum"), "Message Queue"=w869) -> ("error out"=w868:errorcluster)  [unwired: 7 in, 1 out]
      }
      frame "Report" {
        w935 = u16 2 items=["2decimal", "3decimal", "4decimal"] ("Ring")
        w937 = u16 2 items=["2decimal", "3decimal", "4decimal"] ("Ring")
        w939 = u16 0 items=["2decimal", "3decimal", "4decimal"] ("Ring")
        w940 = u16 2 items=["2decimal", "3decimal", "4decimal"] ("Ring")
        n489 = call <vilib>:"Application Directory.vi"() -> ("Application Directory"=w881:path)
        n490 = property on="Varaint Selection" class="Str"() -> ("Value"=w878:string)  [unwired: 2 in, 2 out]
        n491 = local read "Temp value"() -> (w938:dbl[])
        n492 = Build Path(base path=w881, name or relative path=path "Data/Variant_details.ini") -> (appended path=w879:path)
        n493 = local read "Limits"() -> (w943:string[])
        n494 = local read "Voltage health check"() -> (w941:dbl[])
        n495 = local read "weld voltage"() -> (w950:dbl[])
        n496 = call "Float_to_string.vi"("Array"=w938, "Ring"=w939) -> ("Array 2"=w877:string[])  [unwired: 9 in]
        n497 = for {
          tunnel: w943 -> [w972] mode=indexing
          tunnel: [w971] -> w897 mode=indexing
          n498 = Equal?(x=w972, y="NULL") -> (x = y?=w973:bool)
          n499 = case shown="True" w973 {
            tunnel: w972 -> [w975 w977]
            tunnel: [w975 w976] -> w971
            frame False {
            }
            frame True {
              n500 = Concatenate Strings("'" ("string"), w977, "'" ("string")) -> (w976:string)
            }
          }
        }
        n501 = for {
          tunnel: w950 -> [w991] mode=indexing
          tunnel: [w989] -> w917 mode=indexing
          n502 = Multiply(x=w991, y=1000000.0) -> (x*y=w989:dbl)
        }
        n503 = call "temp_selection.vi"("temp_string"=w877, "String"=w878, "configuration file path"=w879) -> ("output array"=w876:string[])  [unwired: 8 in]
        n504 = local read "Result"() -> (w913:bool)
        n505 = call "Float_to_string.vi"("Array"=w941, "Ring"=w940) -> ("Array 2"=w925:string[])  [unwired: 9 in]
        n506 = local read "weld res"() -> (w936:dbl[])
        n507 = call "Faill_adding_value.vi"("index"=12, "input array"=w925, "Boolean"=w913) -> ("output array"=w924:string[])  [unwired: 8 in]
        n508 = call "Float_to_string.vi"("Array"=w936, "Ring"=w937) -> ("Array 2"=w920:string[])  [unwired: 9 in]
        n509 = call "Faill_adding_value.vi"("index"=8, "input array"=w876, "Boolean"=w913) -> ("output array"=w921:string[])  [unwired: 8 in]
        n510 = property on="Tempertaure Sensor" class="Str"() -> ("Value"=w882:string)  [unwired: 2 in, 2 out]
        n511 = Delete From Array(array=w897, length=1, index=29) -> (array with subset deleted=w898:string[])  [unwired: 1 out]
        n512 = Insert Into Array(array=w924, index=12, new element=w921) -> (w955:string[])
        n513 = call "Float_to_string.vi"("Array"=w917, "Ring"=w935) -> ("Array 2"=w915:string[])  [unwired: 9 in]
        n514 = call "Faill_adding_value.vi"("index"=9, "input array"=w920, "Boolean"=w913) -> ("output array"=w918:string[])  [unwired: 8 in]
        n515 = local read "Final Insulation Resistance Result"() -> (w905:string)
        n516 = local read "Final Weld Resistance Result"() -> (w908:string)
        n517 = Insert Into Array(array=w955, index=20, new element=w918) -> (w951:string[])
        n518 = local read "Final Voltage test result"() -> (w907:string)
        n519 = Delete From Array(array=w898, length=1, index=30) -> (array with subset deleted=w896:string[])  [unwired: 1 out]
        n520 = local read "Baseplate to Negative"() -> (w912:string)
        n521 = local read "Baseplate to Positive"() -> (w911:string)
        n522 = call "Faill_adding_value.vi"("index"=9, "input array"=w915, "Boolean"=w913) -> ("output array"=w914:string[])  [unwired: 8 in]
        n523 = local read "final temp result"() -> (w904:string)
        n524 = Insert Into Array(array=w951, index=29, new element=w914) -> (w926:string[])
        n525 = property on="Varaint Selection" class="Str"() -> ("Value"=w886:string)  [unwired: 2 in, 2 out]
        n526 = Replace Array Subset(array=w896, new element=w882, index=28) -> (w888:string[])
        n527 = call "isolation_test_replace_empty.vi"("Isulation test 2"=w905, "Isulation test 1"=w904) -> ("Isulation test 2"=w902:string, "Isulation test 1"=w903:string)  [unwired: 8 in]
        n528 = call "isolation_test_replace_empty.vi"("Isulation test 2"=w907, "Isulation test 1"=w908) -> ("Isulation test 2"=w906:string, "Isulation test 1"=w899:string)  [unwired: 8 in]
        n529 = call "isolation_test_replace_empty.vi"("Isulation test 2"=w911, "Isulation test 1"=w912) -> ("Isulation test 2"=w909:string, "Isulation test 1"=w910:string)  [unwired: 8 in]
        n530 = local read "Result"() -> (w942:bool)
        n531 = Build Array(w903, w902, w899, w906, w910, w909) -> (w949:string[])
        n532 = Concatenate Strings("'" ("string"), w886, "'" ("string")) -> (w885:string)
        n533 = Format Date/Time String(time format string (%c)="%Y-%m-%d") -> (date/time string=w933:string)  [unwired: 2 in]
        n534 = Format Date/Time String(time format string (%c)="%H:%M:%S") -> (date/time string=w932:string)  [unwired: 2 in]
        n535 = local read "Module ID"() -> (w928:string)
        n536 = for {
          tunnel: [w983] -> w948 mode=indexing
          tunnel: w949 -> [w982] mode=indexing
          n537 = Equal?(x=w982, y="NULL") -> (x = y?=w980:bool)
          n538 = case shown="True" w980 {
            tunnel: [w985 w988] -> w983
            tunnel: w982 -> [w984 w988]
            frame False {
              n539 = Concatenate Strings("'" ("string"), w984, "'" ("string")) -> (w985:string)
            }
            frame True {
            }
          }
        }
        n540 = local read "Module Type A/B"() -> (w962:string)
        n541 = Concatenate Strings(w933, "T01" ("string"), w932) -> (w930:string)
        n542 = Insert Into Array(array=w888, index=29, new element=w885) -> (w887:string[])
        n543 = local read "Test Duration"() -> (w964:string)
        n544 = local read "Current"() -> (w953:dbl)
        n545 = Select(t="PASS", s=w942, f="FAIL") -> (s? t:f=w934:string)
        n546 = local read "login"() -> (w963:string)
        n547 = Concatenate Strings(w928, "_" ("string"), w930) -> (w927:string)
        n548 = Build Array(w928, w962, w963, w964, w933, w932, w930, w927, w934) -> (w959:string[])
        n549 = Format Value(format string="%0.3f", value (0)=w953) -> (output string=w901:string)  [unwired: 1 in]
        n550 = local write "Unlock"(TRUE ("Unlock")) -> ()
        n551 = call "isolation_test_replace_empty.vi"("Isulation test 1"=w901) -> ("Isulation test 1"=w900:string)  [unwired: 9 in, 1 out]
        n552 = property on="Start" class="Bool"("Visible"=TRUE) -> ()  [unwired: 2 in, 2 out]
        n553 = Insert Into Array(array=w948, new element #1=w926, new element #2=w900) -> (w945:string[])  [unwired: 1 in]
        n554 = Insert Into Array(array=w945, new element=w887) -> (w944:string[])  [unwired: 1 in]
        n555 = call "Database_C_U.vi"("error in (no error)"=w966, "Basic_info"=w959, "Values"=w944, "Combo Box"="Insert") -> ("error out"=w965:errorcluster)  [unwired: 6 in, 1 out]
        n556 = call-poly "Enqueue Message.vi"("error in (no error)"=w965, "test sequence"=developer_test_sequence."Idle State" ("Enum"), "Message Queue"=w970) -> ("error out"=w891:errorcluster)  [unwired: 7 in, 1 out]
      }
      frame "Error" {
        # "#CodeRecommended - If you ever change the name of this \"Error\" message, you'll need to update the name in the Check Loop Error.vi as well."
        # "#CodeRecommended - Consider creating a system for logging errors in some way. These errors are for notification purposes only. Handling of specific errors should be performed in the message frames that generated the error."
        # "Error - Display an error dialog. This message is sent by the \"Error Handler\" VIs at the end of other loops in this application."
        n557 = Variant To Data(error in=w997, type=errorcluster {"status"=FALSE, "code"=0, "source"=""} ("error constant"), Variant=w996) -> (data=w994:errorcluster, error out=w993:errorcluster)
        n558 = call <vilib>:"Simple Error Handler.vi"("error in (no error)"=w994) -> ()  [unwired: 4 in, 5 out]
        n559 = Merge Errors(w993) -> (w992:errorcluster)
      }
      frame "Confirm Quit" {
        n560 = local write "Unlock"(FALSE ("Unlock")) -> ()
        n561 = local write "stop"(TRUE ("stop")) -> ()
        n562 = call-poly "Enqueue Message.vi"("Priority Message? (F)"=TRUE, "error in (no error)"=w1005, "test sequence"=developer_test_sequence."Exit" ("Enum"), "Message Queue"=w1002) -> ("error out"=w1003:errorcluster)  [unwired: 6 in, 1 out]
        n563 = Merge Errors(w1003) -> (w1004:errorcluster)
      }
      frame "Exit" {
        # "Release the message queue reference"
        # "Exit - Exit the application."
        n564 = disable-structure shown="Disabled" {
          disable-tunnel: w1010 -> [w1017 _]
          frame Disabled {
            n565 = Variant To Data(type=errorcluster {"status"=FALSE, "code"=0, "source"=""} ("error constant"), Variant=w1017) -> (data=w1018:errorcluster)  [unwired: 1 in, 1 out]
            n566 = call <vilib>:"Simple Error Handler.vi"("error in (no error)"=w1018) -> ()  [unwired: 4 in, 5 out]
          }
          frame Enabled {
          }
        }
        n567 = call "Fire User Event - Stop.vi"("User Event - Stop"=w1013) -> ("error out"=w1012:errorcluster)  [unwired: 10 in]
        n568 = Release Queue(queue=w1016, error in (no error)=w1011) -> (error out=w1014:errorcluster)  [unwired: 1 in, 2 out]
        n569 = Merge Errors(w1012, w1014) -> (w1009:errorcluster)
        n570 = call "Main_Vi.vi"("State"="Close") -> ()  [unwired: 9 in, 2 out]
        n571 = local write "Unlock"(FALSE ("Unlock")) -> ()
        n572 = local write "stop"(TRUE ("stop")) -> ()
      }
      frame "Abort" {
      }
    }
    n573 = local read "status_bri"() -> (w93:string)
    n574 = Concatenate Strings(">>>  Executing \"" ("string"), w93, "\"  <<<" ("string")) -> (w92:string)
    n575 = local write "Status Bar"(w92) -> ()
    n576 = call "RMU Error Handler - Message Handling Loop.vi"("error in (no error)"=w97, "Message Queue"=w99) -> ("dup error in"=w98:errorcluster)  [unwired: 8 in, 1 out]
  }
  n577 = flat-sequence {
    frame #0 {
      n578 = local write "stop"(FALSE ("stop")) -> ()
    }
    frame #1 {
      n579 = while {
        i -> [w1029]
        stop <- w1027 stop-if-true
        n580 = local read "reset timer"() -> (w1023:bool)
        n581 = Wait (ms)(milliseconds to wait=u32 500) -> ()  [unwired: 1 out]
        n582 = Equal To 0?(x=w1029) -> (x = 0?=w1026:bool)
        n583 = local read "Unlock"() -> (w1022:bool)
        n584 = local read "Update timer"() -> (w1024:bool)
        n585 = Or(x=w1026, y=w1023) -> (x .or. y?=w1025:bool)
        n586 = case shown="False" w1022 {
          frame False {
          }
          frame True {
            n587 = call "unlock_sol.vi"() -> ()  [unwired: 11 in, 1 out]
          }
        }
        n588 = case shown="True" w1024 {
          tunnel: w1025 -> [_ w1033]
          frame False {
          }
          frame True {
            n589 = call "Elapsed Time"("Reset"=w1033) -> ("Elapsed Time (s)"=→"Elapsed Time (s)":dbl, "Elapsed Time Text"=w1034:string)  [unwired: 11 in, 6 out]
            n590 = String Subset(string=w1034, offset (0)=2) -> (substring=→"Test Duration":string)  [unwired: 1 in]
          }
        }
        n591 = case shown="False" w1023 {
          frame False {
          }
          frame True {
            n592 = local write "reset timer"(FALSE ("reset timer")) -> ()
          }
        }
        n593 = local read "stop"() -> (w1027:bool)
      }
    }
  }
  n594 = while {
    tunnel: w88 -> [w1042]
    shift-right: [w1040] -> w84
    shift-left: w81 -> [w1041]
    tunnel: [w1036] -> w82
    stop <- w1038 stop-if-true
    # "Event Handling Loop"
    n595 = event shown="[4] \"Login Button\": Value Change" {
      selector: w1041 -> [_ _ _ _ _ _]
      dyn-events: [_ _ _ _ _ _] -> w1040
      timeout: _ -> [_ _ _ _ _ _]
      tunnel: [_ _ _ _ _ TRUE ("Discard?")] -> w1038
      tunnel: w1042 -> [w1047 w1051 w1054 w1056 w1058 w1061]
      tunnel: [w1046 _ _ _ _ _] -> w1039
      tunnel: [w1045 w1050 w1053 w1056 w1057 w1061] -> w1037
      event Panel Close? {
        n596 = event-data() -> ()  [unwired: 1 in, 1 out]
        n597 = call-poly "Enqueue Message.vi"("Priority Message? (F)"=TRUE, "test sequence"=developer_test_sequence."Confirm Quit" ("Enum"), "Message Queue"=w1047) -> ("error out"=w1046:errorcluster, "dup Message Queue"=w1045:refnum<queue>)  [unwired: 7 in]
        n598 = event-data("Discard?"=TRUE) -> ()  [unwired: 1 in, 1 out]
      }
      event "Start": Value Change {
        n599 = event-data() -> ()  [unwired: 1 in, 1 out]
        n600 = call-poly "Enqueue Message.vi"("test sequence"=developer_test_sequence."Start Display Board Auto Testing" ("Enum"), "Message Queue"=w1051) -> ("dup Message Queue"=w1050:refnum<queue>)  [unwired: 8 in, 1 out]
        n601 = local write "status_bri"("Start Display Board Auto Testing" ("status_bri")) -> ()
      }
      event "Stop": Value Change {
        n602 = event-data() -> ()  [unwired: 1 in, 1 out]
        n603 = call-poly "Enqueue Message.vi"("test sequence"=developer_test_sequence."Idle State" ("Enum"), "Message Queue"=w1054) -> ("dup Message Queue"=w1053:refnum<queue>)  [unwired: 8 in, 1 out]
      }
      event Application Instance Close {
        n604 = event-data() -> ()  [unwired: 1 in, 1 out]
      }
      event "Login Button": Value Change {
        n605 = event-data() -> ()  [unwired: 1 in, 1 out]
        n606 = call-poly "Enqueue Message.vi"("test sequence"=developer_test_sequence."Admin" ("Enum"), "Message Queue"=w1058) -> ("dup Message Queue"=w1057:refnum<queue>)  [unwired: 8 in, 1 out]
      }
      event User Event {
        (unwired) "\"Exit\" button pressed" ("VI Stopped")
        n607 = event-data() -> ()  [unwired: 1 in, 1 out]
      }
    }
    n608 = call "RMU Error Handler - Event Handling Loop.vi"("error in (no error)"=w1039, "Message Queue"=w1037) -> ("dup error in"=w1036:errorcluster)  [unwired: 8 in, 1 out]
  }
  n609 = Unregister For Events(event registration refnum=w84, error in=w82) -> (error out=w85:errorcluster)
  n610 = Merge Errors(w85, w89) -> (w86:errorcluster)
  n611 = call "Destroy User Event - Stop.vi"("error in (no error)"=w86, "User Event - Stop"=w80) -> ("error out"=w83:errorcluster)  [unwired: 9 in]
  n612 = disable-structure shown="Default" {
    disable-tunnel: w83 -> [_ _]
    frame condition #0 (active) {
    }
    frame condition #1 {
      # "Call Quit LabVIEW if running as a built application."
      n613 = Quit LabVIEW() -> ()  [unwired: 1 in]
    }
  }
